vi "Main_agv.vi"() -> ()   [LabVIEW 2019]
doc: "Self driving example made by ybbaek for ERP42."
uses:
  Ctrl/state.ctl
  Ctrl/agv_config.ctl
  Ctrl/gnss_config.ctl
  <vilib>/userDefined/High Color/IMAQdx.ctl
  Ctrl/system_hw.ctl
  C:/Users/WEGO/Documents/GitHub/Ycar/LabVIEW/Gmap/dll/GMap.NET.WindowsForms.dll
  Gmap/dll/GMap.NET.WindowsForms.dll
  Ctrl/joystick cfg.ctl
  Ctrl/joystick_opval.ctl
  Ctrl/error_cluster.ctl
  Ctrl/imu-cfg.ctl
  Ctrl/ledmatrix_data.ctl
  Ctrl/cmd_common.ctl
  Ctrl/log_buffq.ctl
  Ctrl/agv_cmd_v.ctl
  Ctrl/obstacle_info.ctl
  Ctrl/pid-in-params.ctl
  Ctrl/waypoint_buf.ctl
  Ctrl/cmd_imu.ctl
  Ctrl/gps-databuf.ctl
  Gmap/gmap_fgv-cmd.ctl
  Ctrl/sound-data.ctl
  Subvi/log/logfile-name.vi
  Subvi/global_setting.vi
  Ctrl/pid-cfg.ctl
panel:
  out "mode out":enum16{"joystick", "self-driving"}(ring)
  out "joystick":cluster{"X":dbl, "Y":dbl}[](graph)
  out "Mem":dbl(slide) scale=0.0..16000000000.0 scale format="%_1p"
  out "CPU":dbl(slide) scale=0.0..100.0 scale format="%_1f"
  out "Map_Total":T1(graph)=[{"stop pt array out"=[]}, {"stop pt array out"=[]}, {"stop pt array out"=[{"X"=4530998.623923, "Y"=6178450.805513}, {"X"=4530998.538097, "Y"=6178450.804328}, {"X"=4530998.436351, "Y"=6178450.81696}, {"X"=4530998.335494, "Y"=6178450.839631}, {"X"=4530998.287734, "Y"=6178450.881083}, {"X"=4530998.369203, "Y"=6178451.026592}, {"X"=4530998.616099, "Y"=6178451.104199}, {"X"=4530998.899282, "Y"=6178451.204366}, {"X"=4530999.432829, "Y"=6178451.227778}, {"X"=4530999.994657, "Y"=6178451.1834}, {"X"=4531000.491916, "Y"=6178451.184252}, {"X"=4531000.925496, "Y"=6178451.240374}, {"X"=4531001.380332, "Y"=6178451.342912}, {"X"=4531001.869676, "Y"=6178451.447932}, {"X"=4531002.371383, "Y"=6178451.498979}, {"X"=4531002.905819, "Y"=6178451.53243}, {"X"=4531003.356208, "Y"=6178451.584774}, {"X"=4531003.754389, "Y"=6178451.628375}, {"X"=4531004.172048, "Y"=6178451.698315}, {"X"=4531004.577345, "Y"=6178451.822228}, {"X"=4531004.966722, "Y"=6178451.959958}, {"X"=4531005.304781, "Y"=6178452.098985}, {"X"=4531005.558793, "Y"=6178452.256904}, {"X"=4531005.663298, "Y"=6178452.468907}, {"X"=4531005.735073, "Y"=6178452.698506}, {"X"=4531005.808628, "Y"=6178452.948183}, {"X"=4531005.871598, "Y"=6178453.271912}, {"X"=4531005.874357, "Y"=6178453.496547}, {"X"=4531005.809877, "Y"=6178453.736296}, {"X"=4531005.695859, "Y"=6178453.997419}, {"X"=4531005.514602, "Y"=6178454.273656}, {"X"=4531005.263439, "Y"=6178454.53489}, {"X"=4531004.89372, "Y"=6178454.812535}, {"X"=4531004.439065, "Y"=6178455.099032}, {"X"=4531003.810977, "Y"=6178455.363081}, {"X"=4531003.261601, "Y"=6178455.548003}, {"X"=4531002.709556, "Y"=6178455.702809}, {"X"=4531002.017699, "Y"=6178455.827609}, {"X"=4531001.45765, "Y"=6178455.892064}, {"X"=4531000.845393, "Y"=6178455.947777}, {"X"=4531000.166788, "Y"=6178456.028643}, {"X"=4530999.390883, "Y"=6178456.172335}, {"X"=4530998.64593, "Y"=6178456.278353}, {"X"=4530997.881499, "Y"=6178456.358033}, {"X"=4530997.114399, "Y"=6178456.407596}, {"X"=4530996.505611, "Y"=6178456.308947}, {"X"=4530996.309053, "Y"=6178456.025486}, {"X"=4530996.530954, "Y"=6178455.627487}, {"X"=4530996.701536, "Y"=6178455.230783}, {"X"=4530996.904848, "Y"=6178454.816484}, {"X"=4530997.126748, "Y"=6178454.418484}, {"X"=4530997.382268, "Y"=6178454.012928}, {"X"=4530997.604168, "Y"=6178453.614928}, {"X"=4530997.677451, "Y"=6178453.281051}, {"X"=4530997.953338, "Y"=6178452.911871}, {"X"=4530998.350449, "Y"=6178452.556397}, {"X"=4530998.886482, "Y"=6178452.22089}, {"X"=4530999.254422, "Y"=6178451.923168}, {"X"=4530999.465739, "Y"=6178451.599218}, {"X"=4530999.52666, "Y"=6178451.319314}, {"X"=4530999.555832, "Y"=6178451.261562}, {"X"=4530999.57442, "Y"=6178451.277862}, {"X"=4530999.57531, "Y"=6178451.287901}, {"X"=4530999.561169, "Y"=6178451.321796}, {"X"=4530999.562948, "Y"=6178451.341874}, {"X"=4530999.582425, "Y"=6178451.368212}, {"X"=4530999.584204, "Y"=6178451.38829}, {"X"=4530999.552364, "Y"=6178451.415925}, {"X"=4530999.520524, "Y"=6178451.44356}]}]
  out "Error cluster out":T2
  out "State":T3
  out "loop count out":T4
  out "Time info":T5={"Time_total"=2.602255344390869, "Time_run"=0.0, "Time_wait"=2.602255344390869} {"Time_total" format="%.1f"; "Time_run" format="%.1f"; "Time_wait" format="%.1f"}
  in  "ybbaek copyright":string="Made by ybbaek"
  in  "Tab_main":enum32{"Main UI", "Config"}(tab)
  in  "sel driving mode":bool
  out "point all":T6(graph)
  out "Image_color":T7(plugin-control)
  out "LiDAR Display":T8(graph)=[{"Array out"=[{"x"=0.0, "y"=0.0}, {"x"=1.1593565889372284, "y"=0.6693548387096749}, {"x"=0.0, "y"=0.0}, {"x"=-1.0549176217638336, "y"=0.8241919750327333}]}, {"Array out"=[{"x"=0.2522907528348065, "y"=-0.9679098297538085}, {"x"=0.24254936669439534, "y"=-0.9773529581047719}, {"x"=0.2311466414632541, "y"=-0.9780573756893088}, {"x"=0.22013509908304701, "y"=-0.9790570913647973}, {"x"=0.21252085784239536, "y"=-0.9958252595118947}, {"x"=0.20354094471094616, "y"=-1.0117287600074318}, {"x"=0.19216973869870496, "y"=-1.0136956417132665}, {"x"=0.18000768331848416, "y"=-1.0144024331823698}, {"x"=0.16839887138747095, "y"=-1.0130996101644822}, {"x"=0.13425505056226478, "y"=-1.0262556121154827}, {"x"=0.1235875841313941, "y"=-1.0321271041148787}, {"x"=0.11209282841873203, "y"=-1.0392221900619176}, {"x"=0.05343374521033363, "y"=-1.046887241957221}, {"x"=0.04042794561687843, "y"=-1.043467126321284}, {"x"=0.029222649738115388, "y"=-1.0400895570777948}, {"x"=0.017036653056079584, "y"=-1.0411106160983312}, {"x"=0.005134519873165823, "y"=-1.0459873979669507}, {"x"=-0.006314508810403322, "y"=-1.052481057776568}, {"x"=-0.0010110708384152129, "y"=0.0007350073194916896}, {"x"=0.001141793129326704, "y"=-0.000508732198531145}, {"x"=3.2663755682368802, "y"=-0.2409423369298104}, {"x"=3.2682974720954157, "y"=-0.3156008299968731}, {"x"=0.2578445921202276, "y"=-0.9633398822919943}, {"x"=0.24825106355708415, "y"=-0.9697280079706766}, {"x"=0.23807482826060586, "y"=-0.978709833734536}, {"x"=0.2259487186744975, "y"=-0.977475185889316}, {"x"=0.21158377943464465, "y"=-1.0172282459114828}, {"x"=0.19914944525971545, "y"=-1.0156596371091782}, {"x"=0.1865928320916569, "y"=-1.0144828066616085}, {"x"=0.17483503646380183, "y"=-1.0125161529697693}, {"x"=0.16287079283932476, "y"=-1.0140030102716113}, {"x"=0.12952794839316292, "y"=-1.0293827085127565}, {"x"=0.11787284633583305, "y"=-1.0345566947232467}, {"x"=0.10740206219988796, "y"=-1.0409740856693848}, {"x"=0.059584119729109916, "y"=-1.0493096457557736}, {"x"=0.047185684852639714, "y"=-1.0479382191450923}, {"x"=0.034928532242850446, "y"=-1.0409141403763138}, {"x"=0.022959984335812273, "y"=-1.0392464044293341}, {"x"=0.011371685382685006, "y"=-1.0424379764626561}, {"x"=-0.000572277070893853, "y"=-1.0492498439356348}, {"x"=-0.012356443381401225, "y"=-1.0536775506799803}]}, {"Array out"=[]}, {"Array out"=[]}, {"Array out"=[]}]
  out "Pid dt":u32=100
  out "heaading_ui":dbl
  out "Distance_left":dbl format="%.1f"
  out "Dis_gap":dbl format="%.1f"
  out "pro_all":u8(slide) scale=0.0..100.0
  out "pro_curr":dbl(slide)=nan scale=0.0..1.0
  out "stop time":dbl(slide)=2.7272372245788574 scale=0.0..5.0
  in  "gmap zoom":dbl(slide) scale=3.0..20.0
  in  "GMapControl":refnum<k24>(container)
  out "Map_Current":T9(graph)=[{"heading_curr "=[]}, {"heading_curr "=[]}, {"heading_curr "=[{"x"=0.0, "y"=0.0}, {"x"=0.0, "y"=0.0}, {"x"=0.0, "y"=0.0}, {"x"=0.0, "y"=0.0}, {"x"=0.0, "y"=0.0}, {"x"=0.0, "y"=0.0}]}, {"heading_curr "=[]}, {"heading_curr "=[{"x"=0.0, "y"=0.0}, {"x"=0.0, "y"=0.0}]}, {"heading_curr "=[{"x"=0.0, "y"=0.0}, {"x"=0.0, "y"=0.0}]}, {"heading_curr "=[{"x"=0.0, "y"=0.0}, {"x"=3.6739403974420594e-16, "y"=6.0}]}, {"heading_curr "=[{"x"=0.0, "y"=0.0}, {"x"=3.6739403974420594e-16, "y"=6.0}]}]
  in  "imu reset M":bool
  out "latlong_Gmap":cluster{dbl, dbl} {"?" format="%.8f"; "?" format="%.8f"}
  out "latlong_GNSS":cluster{dbl, dbl} {"?" format="%.8f"; "?" format="%.8f"}
  in  "SetMapProvider":u16(ring)=12 items=["None", "OpenStreetMap", "OpenStreet4UMap", "OpenCycleMap", "OpenCycleLandscapeMap", "OpenCycleTransportMap", "OpenStreetMapQuest", "OpenStreetMapQuestSattelite", "OpenStreetMapQuestHybrid", "OpenSeaMapHybrid", "WikiMapiaMap", "BingMap", "BingSatelliteMap", "BingHybridMap", "YahooMap", "YahooSatelliteMap", "YahooHybridMap", "GoogleMap", "GoogleSatelliteMap", "GoogleHybridMap", "GoogleTerrainMap", "GoogleChinaMap", "GoogleChinaSatelliteMap", "GoogleChinaHybridMap", "GoogleChinaTerrainMap", "GoogleKoreaMap", "GoogleKoreaSatelliteMap", "GoogleKoreaHybridMap", "NearMap", "NearSatelliteMap", "NearHybridMap", "OviMap", "OviSatelliteMap", "OviHybridMap", "OviTerrainMap", "YandexMap", "YandexSatelliteMap", "YandexHybridMap", "LithuaniaMap", "Lithuania 2.5d Map", "LithuaniaOrtoFotoMap", "LithuaniaOrtoFotoMapOld", "LithuaniaHybridMap", "LithuaniaHybridMapOld", "LithuaniaTOP50", "LatviaMap", "MapBender, WMS demo", "TurkeyMap", "CloudMade, Demo", "SpainMap", "CzechMap", "CzechSatelliteMap", "CzechHybridMap", "CzechTuristMap", "CzechHistoryMap", "ArcGIS_Imagery_World_2D_Map", "ArcGIS_ShadedRelief_World_2D_Map", "ArcGIS_StreetMap_World_2D_Map", "ArcGIS_Topo_US_2D_Map", "ArcGIS_World_Physical_Map", "ArcGIS_World_Shaded_Relief_Map", "ArcGIS_World_Street_Map", "ArcGIS_World_Terrain_Base_Map", "ArcGIS_World_Topo_Map", "ArcGIS_DarbAE_Q2_2011_NAVTQ_Eng_V5_MapProvider"]
  in  "PinDropMrkr":T10(ring)=enum."red_dot" caption="Pin Drop Marker"
  in  "zoom-center":bool
  in  "Zoom":bool
  in  "Scale_map":dbl(slide)=5.0 min=0.0 scale=5.0..100.0
  in  "ratio":dbl=10.0 format="%#_13g"
  in  "full scale":bool
  out "Steer_PID2":T11(graph)={"output high"=42.0, "output low"=10.0, "output"=0.0}
  in  "Speed":dbl(slide)=33.0 min=0.0 max=255.0 scale=0.0..255.0
  in  "set state value":T3
  in  "state change":bool
  out "network check":bool
  in  "Tap_config":T12(tab)=enum."GNSS Gmap"
  out "Mem usage":dbl(slide) scale=0.0..20000.0 scale format="%_1f"
  out "CPU Usage":dbl(slide) scale=0.0..100.0 scale format="%_1f"
  out "Mem Usage 2":string
  in  "HW info":T13={"AGV"=enum."Ycar", "Lidar 1"=enum."RPLidar A2", "Lidar 2"=enum."none", "GPS"=enum."none", "Camera"=enum."MS LifeCam", "Joystick"=enum."joystick", "sound"=enum."none", "IMU"=enum."none", "Led"=enum."none"}
  out "CPU Chart":dbl(graph)
  out "Mem  Chart":dbl(graph)
  in  "AGV-2":enum32{"Status"}(tab)
  out "batt":dbl(slide) scale=26.0..29.0
  out "AGV velocity Chart":T14(graph)
  out "System Feedback":T15
  in  "AGV cfg":T16={"Port"="COM6", "limits"={"speed limits"={"max"=100.0, "min"=0.0}, "steer limits"={"width"=40.0, "offset"=8.0}}, "dir"=FALSE}
  in  "Lookahead cfg":T17={"lookahead points"=64.0, "lookahead distance"=2.0} {"lookahead distance" format="%.1f"; "lookahead points" format="%#_13g"}
  in  "State machine cfg":T18={" turn steer speed"=0.0, "move speed"=0.0, "slow down factor"=1.0, "adjust angle margin"=0.0} {"slow down factor" min=1.0}
  out "Slide":cluster{dbl, dbl, dbl}(slide) scale=0.0..1.0
  out "Stop point count":u32(slide) scale=-1.0..60.0
  in  "Tab_Lidar-config":enum32{"VLP16", "Tim571", "RPLiar A123"}(tab)=enum."RPLiar A123"
  in  "TIM571 cfg":T19 {"h range" scale=-180.0..180.0}
  in  "RPLidar cfg":T20={"port"="COM3", "dt"=4, "cicle"=28, "speed"=500, "rate"=115200} {"speed" scale=100.0..1000.0}
  out "LiDAR Display for cfg":T8(graph)=[{"Array out"=[{"x"=0.0, "y"=0.0}, {"x"=0.7193398003386512, "y"=0.6946583704589973}, {"x"=0.0, "y"=0.0}, {"x"=-0.9271838545667873, "y"=0.37460659341591224}]}, {"Array out"=[]}, {"Array out"=[]}, {"Array out"=[]}, {"Array out"=[]}]
  in  "lidat setting tab":enum32{"Range", "Limit", "Graph"}(tab)
  in  "VLP16 cfg":T21={"h range"={46, -68}, "v range"={8, -4}} {"v range" scale=-15.0..15.0; "h range" scale=-180.0..180.0}
  in  "Obstacle limit cfg":cluster{"Range":dbl, "Points":u16}={"Range"=1.0, "Points"=110} {"Points" min=10 max=5000 scale=10.0..100.0; "Range" min=0.5 max=200.0 scale=0.5..20.0}
  in  "Lidar graph scale":dbl(slide)=1.0 min=1.0 scale=1.0..10.0
  in  "PID cfg":T22={"PID gains"={"proportional gain (Kc)"=0.01, "integral time (Ti, min)"=0.0, "derivative time (Td, min)"=0.0}, "PID limits"={"output high"=40.0, "output low"=15.0}, "dt_pid"=100} {"PID limits"."output low" format="%.3f"; "PID limits"."output high" format="%.3f"; "PID gains"."derivative time (Td, min)" format="%.4f"; "PID gains"."integral time (Ti, min)" format="%.4f"; "PID gains"."proportional gain (Kc)" format="%.4f"}
  out "Steer_PID1":T11(graph)={"output high"=40.0, "output low"=15.0, "output"=0.0}
  out "Image_binary 2":T7(plugin-control)
  in  "GNSS cfg":T23={"Port"="COM10", "heading select"="", "PwrPak7_mode select"=[], "rate"=115200}
  in  "gmap-dt2":u32=1000
  in  "gmap-dt1":u32=200
  out "Lon_GM":dbl format="%.9f"
  out "Lat_GM":dbl format="%.9f"
  out "Lat_DbClk":dbl format="%.9f"
  out "Lon_DbClk":dbl format="%.9f"
  out "Image_binary":T7(plugin-control)
  out "Image_gray":T7(plugin-control)
  in  "Tab vision-setting":enum32{"Port ", "Config", "camera attrib"}(tab)
  in  "camera cfg":cluster{"Port":T24, "Camera file":path}={"Port"="cam1", "Camera file"=path "C:/AGV/Config/camera/MS_LifeCam_30fps_160x120.icd"}
  in  "Vison cfg":T25 {"Threshold Range"."Upper value" scale=0.0..255.0; "Threshold Range"."Lower value" scale=0.0..255.0}
  in  "camera_attrib":cluster{"brightness":u16, "ExposureTimeAbs":dbl}={"brightness"=0, "ExposureTimeAbs"=15000.0} {"brightness" scale=0.0..10.0; "ExposureTimeAbs" scale=0.0..30000.0}
  in  "IMU cfg":T26={"Port"="COM10", "offset"=0.0, "rate"=115200}
  out "IMU out":T27 {"gyr" format="%.2f"; "mag" format="%.2f"; "acc" format="%.2f"; "angle" format="%.2f"}
  out "dir":picture
  out "heading_cfg":dbl format="%.1f"
  in  "imu reset":bool
  out "ang":dbl[](array[numeric])
  out "Deg-gap_heading-wpt":dbl format="%.1f"
  in  "config save":bool
  in  "config load":bool
  in  "config_file-name":string="user1"
  out "error out":errorcluster
  out "log path":string
  in  "waypoint files cfg":T28={"Waypoint array"=[{"sel"=TRUE, "inv"=FALSE, "path"=path "C:/AGV/Config/waypoint/wpt_shinsung-circle_20201004-1.txt"}]}
  out "Total map cfg":T29(graph)=[{"ref waypt 0703 A \ngoal point start"=[]}, {"ref waypt 0703 A \ngoal point start"=[{"X"=4530998.623923, "Y"=6178450.805513}, {"X"=4530998.538097, "Y"=6178450.804328}, {"X"=4530998.436351, "Y"=6178450.81696}, {"X"=4530998.335494, "Y"=6178450.839631}, {"X"=4530998.287734, "Y"=6178450.881083}, {"X"=4530998.369203, "Y"=6178451.026592}, {"X"=4530998.616099, "Y"=6178451.104199}, {"X"=4530998.899282, "Y"=6178451.204366}, {"X"=4530999.432829, "Y"=6178451.227778}, {"X"=4530999.994657, "Y"=6178451.1834}, {"X"=4531000.491916, "Y"=6178451.184252}, {"X"=4531000.925496, "Y"=6178451.240374}, {"X"=4531001.380332, "Y"=6178451.342912}, {"X"=4531001.869676, "Y"=6178451.447932}, {"X"=4531002.371383, "Y"=6178451.498979}, {"X"=4531002.905819, "Y"=6178451.53243}, {"X"=4531003.356208, "Y"=6178451.584774}, {"X"=4531003.754389, "Y"=6178451.628375}, {"X"=4531004.172048, "Y"=6178451.698315}, {"X"=4531004.577345, "Y"=6178451.822228}, {"X"=4531004.966722, "Y"=6178451.959958}, {"X"=4531005.304781, "Y"=6178452.098985}, {"X"=4531005.558793, "Y"=6178452.256904}, {"X"=4531005.663298, "Y"=6178452.468907}, {"X"=4531005.735073, "Y"=6178452.698506}, {"X"=4531005.808628, "Y"=6178452.948183}, {"X"=4531005.871598, "Y"=6178453.271912}, {"X"=4531005.874357, "Y"=6178453.496547}, {"X"=4531005.809877, "Y"=6178453.736296}, {"X"=4531005.695859, "Y"=6178453.997419}, {"X"=4531005.514602, "Y"=6178454.273656}, {"X"=4531005.263439, "Y"=6178454.53489}, {"X"=4531004.89372, "Y"=6178454.812535}, {"X"=4531004.439065, "Y"=6178455.099032}, {"X"=4531003.810977, "Y"=6178455.363081}, {"X"=4531003.261601, "Y"=6178455.548003}, {"X"=4531002.709556, "Y"=6178455.702809}, {"X"=4531002.017699, "Y"=6178455.827609}, {"X"=4531001.45765, "Y"=6178455.892064}, {"X"=4531000.845393, "Y"=6178455.947777}, {"X"=4531000.166788, "Y"=6178456.028643}, {"X"=4530999.390883, "Y"=6178456.172335}, {"X"=4530998.64593, "Y"=6178456.278353}, {"X"=4530997.881499, "Y"=6178456.358033}, {"X"=4530997.114399, "Y"=6178456.407596}, {"X"=4530996.505611, "Y"=6178456.308947}, {"X"=4530996.309053, "Y"=6178456.025486}, {"X"=4530996.530954, "Y"=6178455.627487}, {"X"=4530996.701536, "Y"=6178455.230783}, {"X"=4530996.904848, "Y"=6178454.816484}, {"X"=4530997.126748, "Y"=6178454.418484}, {"X"=4530997.382268, "Y"=6178454.012928}, {"X"=4530997.604168, "Y"=6178453.614928}, {"X"=4530997.677451, "Y"=6178453.281051}, {"X"=4530997.953338, "Y"=6178452.911871}, {"X"=4530998.350449, "Y"=6178452.556397}, {"X"=4530998.886482, "Y"=6178452.22089}, {"X"=4530999.254422, "Y"=6178451.923168}, {"X"=4530999.465739, "Y"=6178451.599218}, {"X"=4530999.52666, "Y"=6178451.319314}, {"X"=4530999.555832, "Y"=6178451.261562}, {"X"=4530999.57442, "Y"=6178451.277862}, {"X"=4530999.57531, "Y"=6178451.287901}, {"X"=4530999.561169, "Y"=6178451.321796}, {"X"=4530999.562948, "Y"=6178451.341874}, {"X"=4530999.582425, "Y"=6178451.368212}, {"X"=4530999.584204, "Y"=6178451.38829}, {"X"=4530999.552364, "Y"=6178451.415925}, {"X"=4530999.520524, "Y"=6178451.44356}]}]
  in  "test waypoint":bool
  in  "stop points edit":bool
  in  "stop point config":cluster{"distance":dbl, "time":dbl}={"distance"=1.0, "time"=5.0}
  in  "Joystick cfg":T30={"Type"=enum."Logitech F710", "steer limit"={"min"=10.0, "max"=42.0, "scale"=0.0, "offset"=0.0}, "speed limit"={"min"=10.0, "max"=42.0, "pwm max"=0.0}, "ID"=0, "joystick max"=0.0}
  out "opval":T31
  out "pid limit ref":cluster{dbl, dbl}
  out "receive buff out":string
  in  "sound cfg":T32={"id"=0, "music folder"=path "C:/AGV/Config/sound/music", "engine"=path "C:/AGV/Config/sound/lock.wav", "warning"=path "C:/AGV/Config/sound/lock.wav", "msg"=path "C:/AGV/Config/sound/lock.wav", "music"=path "C:/AGV/Config/sound/lock.wav", "unlock"=path "C:/AGV/Config/sound/lock.wav"}
  in  "ledmatrix cfg":T33={"ip"="", "data"="", "Port"="COM6", "time"=""}
  out "LiDAR img":T7(plugin-control)
  in  "pause-resume":bool
  in  "Checking":bool
  in  "start-stop":bool
  in  "close":bool
  in  "Status detail":string="\r\n00:38:31.5 - System start \r\n"
  # "Status main"
  # "64\n  5"
  # "254\n     0"
  # "40\n  8"
  # "4\n44\n444"
  # "X, Y, Z / roll, pitch, yaw"
  # "<Xbox>\njoy max: 32767\nsteer min 10 / scale 16\nsteer max 42 / offset 26\nspeed min 10 / pwm max 255\nspeed max 200"
  # "<F710>\njoy max: 32767\nsteer min 10 / scale 20 (-20)\nsteer max 42 / offset 30\nspeed min 10 / pwm max 255\nspeed max 200              -255"
  # "SRC (Self driving RC Car)"
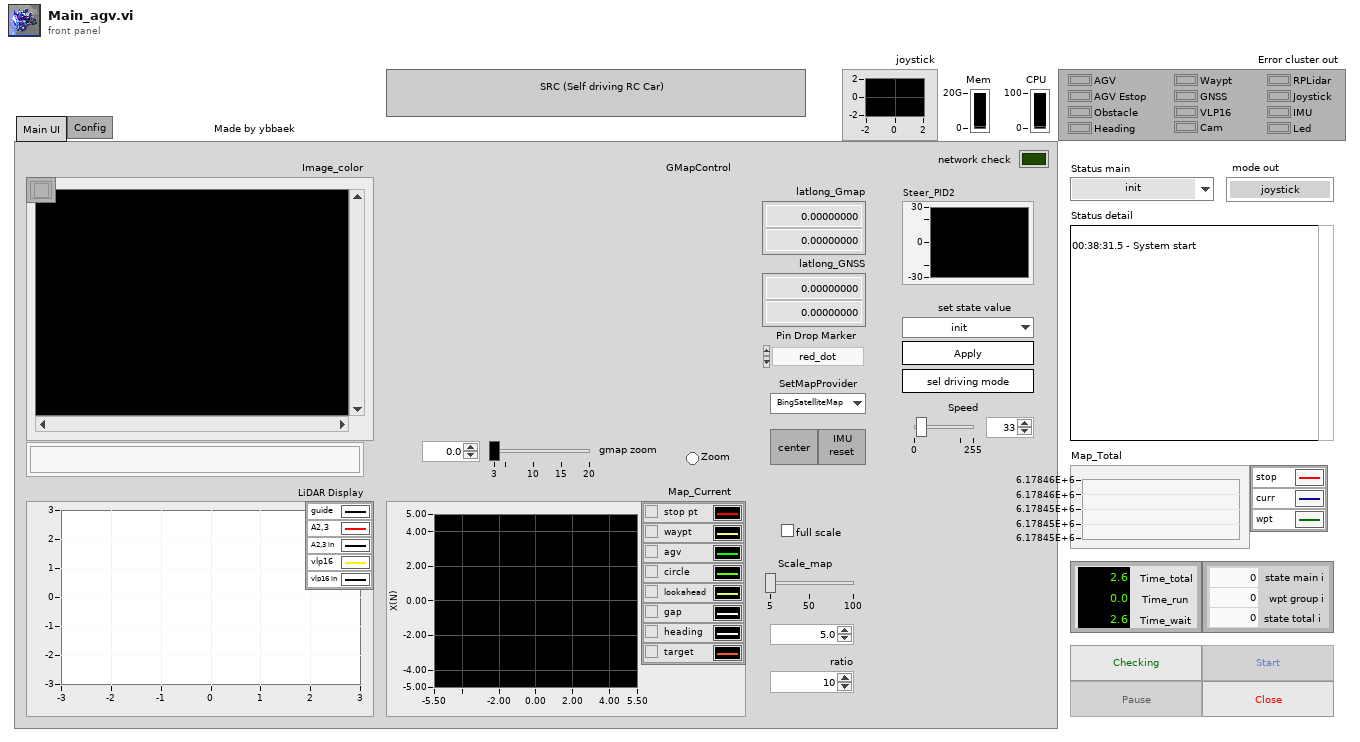
[diagram p1: front panel]
types:
  T1 = cluster{"stop pt array out":cluster{"X":dbl, "Y":dbl}[]}[]
  T2 = typedef "error_cluster.ctl" = cluster{"AGV":u8, "AGV Estop":u8, "Obstacle":u8, "Heading":u8, "Waypt":u8, "GNSS":u8, "VLP16":u8, "Cam":u8, "RPLidar":u8, "Joystick":u8, "IMU":u8, "Led":u8}
  T3 = typedef "state.ctl" = enum16{"init", "Test circular track", "start point", "start heading adjust", "wait before start", "stop point check", "stop point start", "end point", "entering ending point", "move", "move heading adjust"}
  T4 = cluster{"wpt group i":i32, "state total i":i32, "state main i":i32}
  T5 = cluster{"Time_total":dbl, "Time_run":dbl, "Time_wait":dbl}
  T6 = cluster{"Points-2":cluster{"X":sgl, "Y":sgl}[]}[]
  T7 = typedef "IMAQ Image.ctl" = refnum<image>
  T8 = cluster{"Array out":cluster{"x":dbl, "y":dbl}[]}[]
  T9 = cluster{"heading_curr ":cluster{"x":dbl, "y":dbl}[]}[]
  T10 = enum16{"none", "arrow", "blue", "blue_small", "blue_dot", "blue_pushpin", "brown_small", "gray_small", "green", "green_small", "green_dot", "green_pushpin", "green_big_go", "yellow", "yellow_small", "yellow_dot", "yellow_big_pause", "yellow_pushpin", "lightblue", "lightblue_dot", "lightblue_pushpin", "orange", "orange_small", "orange_dot", "pink", "pink_dot", "pink_pushpin", "purple", "purple_small", "purple_dot", "purple_pushpin", "red", "red_small", "red_dot", "red_pushpin", "red_big_stop", "black_small", "white_small"}
  T11 = cluster{"output high":dbl, "output low":dbl, "output":dbl}
  T12 = enum32{"System", "AGV", "LIDAR", "PID", "GNSS Gmap", "Vision", "IMU", "File", "Waypoint", "Joystick", "Network", "Sound", "Led display", "Etc"}
  T13 = typedef "system_hw.ctl" = cluster{"AGV":enum16{"none", "ERP42", "Scout", "Ycar"}, "Lidar 1":enum16{"none", "VLP16", "TIM571", "RPLidar A2", "RPLidar A3"}, "Lidar 2":enum16{"none", "VLP16", "TIM571", "RPLidar A2", "RPLidar A3"}, "GPS":enum16{"none", "F9P", "M8P", "PwrPak7", "19X HVS"}, "Camera":enum16{"none", "C920", "C922", "GT1290C", "MS LifeCam"}, "Joystick":enum16{"none", "joystick"}, "sound":enum16{"none", "speaker"}, "IMU":enum16{"none", "MW-AHRSv1"}, "Led":enum16{"none", "LedMatrix 8x32"}}
  T14 = cluster{"Linear Velocity (m/s)":dbl, "Angular Velocity (rad/s)":dbl, "Battery Voltage":dbl}
  T15 = cluster{"state":string, "Mode":u8, "Battery V":dbl, "error High":u8, "error Low":u8}
  T16 = typedef "agv_config.ctl" = cluster{"Port":refnum<visa-resource-name>, "limits":cluster{"speed limits":cluster{"max":dbl, "min":dbl}, "steer limits":cluster{"width":dbl, "offset":dbl}}, "dir":bool}
  T17 = cluster{"lookahead points":dbl, "lookahead distance":dbl}
  T18 = cluster{" turn steer speed":dbl, "move speed":dbl, "slow down factor":dbl, "adjust angle margin":dbl}
  T19 = cluster{"TIM571 IP":string, "h range":cluster{i16, i16}}
  T20 = cluster{"port":refnum<visa-resource-name>, "dt":u32, "cicle":u8, "speed":u16, "rate":u32}
  T21 = cluster{"h range":cluster{i16, i16}, "v range":cluster{i8, i8}}
  T22 = cluster{"PID gains":cluster{"proportional gain (Kc)":dbl, "integral time (Ti, min)":dbl, "derivative time (Td, min)":dbl}, "PID limits":cluster{"output high":dbl, "output low":dbl}, "dt_pid":u32}
  T23 = typedef "gnss_config.ctl" = cluster{"Port":refnum<visa-resource-name>, "heading select":string, "PwrPak7_mode select":string[], "rate":u32}
  T24 = typedef "IMAQdx.ctl" = refnum<k21>
  T25 = cluster{"Clamp Settings":cluster{"Contrast":i32, "Filter width":i32, "Steepness":i32, "Subsampling Ratio":u32, "Show Search Area":bool, "Show Search Lines":bool, "Show Edges Found":bool, "Show Result":bool}, "Threshold Range":cluster{"Lower value":sgl, "Upper value":sgl}, "N of Erosion 1":i32, "N of Erosion 2":i32}
  T26 = typedef "imu-cfg.ctl" = cluster{"Port":refnum<visa-resource-name>, "offset":dbl, "rate":u32}
  T27 = cluster{"angle":dbl[], "acc":dbl[], "mag":dbl[], "gyr":dbl[]}
  T28 = cluster{"Waypoint array":cluster{"sel":bool, "inv":bool, "path":path}[]}
  T29 = cluster{"ref waypt 0703 A \ngoal point start":cluster{"X":dbl, "Y":dbl}[]}[]
  T30 = typedef "joystick cfg.ctl" = cluster{"Type":enum16{"Logitech F710", "Xbox"}, "steer limit":cluster{"min":dbl, "max":dbl, "scale":dbl, "offset":dbl}, "speed limit":cluster{"min":dbl, "max":dbl, "pwm max":dbl}, "ID":i32, "joystick max":dbl}
  T31 = typedef "joystick_opval.ctl" = cluster{"curr":u32, "last":u32}
  T32 = cluster{"id":u32, "music folder":path, "engine":path, "warning":path, "msg":path, "music":path, "unlock":path}
  T33 = typedef "ledmatrix_data.ctl" = cluster{"ip":string, "data":string, "Port":refnum<visa-resource-name>, "time":string}
  T34 = cluster{"VLP16 cfg":refnum<vi>, "TIM571 cfg":refnum<vi>, "PID cfg":refnum<vi>, "AGV cfg":refnum<vi>, "GNSS cfg":refnum<vi>, "camera cfg":refnum<vi>, "ybbaek copyright":refnum<vi>, "Obstacle limit cfg":refnum<vi>, "State machine cfg":refnum<vi>, "Lookahead cfg":refnum<vi>, "waypoint files cfg":refnum<vi>, "Vison cfg":refnum<vi>, "RPLidar cfg":refnum<vi>, "point all":refnum<vi>, "HW info":refnum<vi>, "Joystick cfg":refnum<vi>, "GMapControl":refnum<vi>, "IMU cfg":refnum<vi>, "ledmatrix cfg":refnum<vi>}
  T35 = enum16{"Config Save", "Config Load", "LastRUN Save", "LastRUN Load"}
  T36 = typedef "cmd_common.ctl" = enum16{"read", "write"}
  T37 = cluster{"Name":string, "Color":u32, "Style":u8, "Point Style":u8, "Name Visible":bool, "Allow Drag":bool, "Annotation Mode":u32, "Plot":i32, "Index":i32, "Position":cluster{"X":dbl, "Y":dbl}, "X Scale":u32, "Y Scale":u32, "Show Arrow":bool, "Lock Name":bool, "Plot Area":i32, "Label Offset":cluster{"X":dbl, "Y":dbl}}
  T38 = enum8{"Enabled", "Disabled", "Disabled and Grayed Out"}
  T39 = typedef "log_buffq.ctl" = enum16{"create", "write", "read", "close"}
  T40 = typedef "agv_cmd_v.ctl" = enum16{"write limit", "init stop", "write", "read"}
  T41 = cluster{"zoom":dbl, "dt clear":u32, "dt add ":u32, "PinDropMrkr":enum16{"none", "arrow", "blue", "blue_small", "blue_dot", "blue_pushpin", "brown_small", "gray_small", "green", "green_small", "green_dot", "green_pushpin", "green_big_go", "yellow", "yellow_small", "yellow_dot", "yellow_big_pause", "yellow_pushpin", "lightblue", "lightblue_dot", "lightblue_pushpin", "orange", "orange_small", "orange_dot", "pink", "pink_dot", "pink_pushpin", "purple", "purple_small", "purple_dot", "purple_pushpin", "red", "red_small", "red_dot", "red_pushpin", "red_big_stop", "black_small", "white_small"}, "zoom n center":bool}
  T42 = cluster{"VLP16 cfg":cluster{"h range":cluster{i16, i16}, "v range":cluster{i8, i8}}, "TIM571 cfg":cluster{"IP":string, "h range":cluster{i16, i16}}, "AGV cfg":T16, "GPS cfg":cluster{"Port":refnum<visa-resource-name>, "heading select":string, "PwrPak7_mode select":string[], "rate":u32}, "PID cfg":cluster{"PID gains":cluster{"proportional gain (Kc)":dbl, "integral time (Ti, min)":dbl, "derivative time (Td, min)":dbl}, "PID limits":cluster{"output high":dbl, "output low":dbl}, "dt pid":u32}, "Lookahead cfg":cluster{"lookahead pts n":dbl, "lookahead distance":dbl}, "Obstacle limit range":cluster{"RL range":dbl, "Point limit":u16}, "State machine parameter":cluster{"angle adjust limit":dbl}, "waypoint group":cluster{"Waypoint array":cluster{"sel":bool, "inv":bool, "path":path}[]}, "State machine cfg":cluster{" turn angular speed":dbl, "move linear speed":dbl, "decrease factor linear speed":dbl, "adjust angle margin":dbl}, "camera cfg":cluster{"Port":T24, "Camera file":path}, "ROI-clamp":cluster{"Global Rectangle":i32[], "Contours":cluster{"Contour Type":u32, "ROI Type":u32, "Points":i32[]}[]}, "x-center":dbl, "Image Size":cluster{"x":i32, "y":i32}, "Angle deg":sgl, "Vison cfg":cluster{"Clamp Settings":cluster{"Contrast":i32, "Filter width":i32, "Steepness":i32, "Subsampling Ratio":u32, "Show Search Area":bool, "Show Search Lines":bool, "Show Edges Found":bool, "Show Result":bool}, "Range":cluster{"Lower value":sgl, "Upper value":sgl}, "N of Erosion 1":i32, "N of Erosion 2":i32}, "RPLidar cfg":cluster{"port":refnum<visa-resource-name>, "dt":u32, "update":u8, "speed":u16, "rate ":u32}, "HW info":T13, "Joystick cfg":T30, "IMU cfg":T26, "ledmatrix cfg":T33}
  T43 = cluster{"Name":string, "Color":u32, "Style":u8, "Point Style":u8, "Name Visible":bool, "Allow Drag":bool, "Annotation Mode":u32, "Plot":i32, "Index":i32, "Position":cluster{"X":dbl, "Y":dbl}, "X Scale":u32, "Y Scale":u32, "Show Arrow":bool, "Lock Name":bool, "Plot Area":i32, "Label Offset":cluster{"X":dbl, "Y":dbl}}[]
  T44 = cluster{"Global Rectangle":i32[], "Contours":cluster{"Contour Type":u32, "ROI Type":u32, "Points":i32[]}[]}
  T45 = cluster{"Lat_GM":refnum<vi>, "Lon_GM":refnum<vi>, "Lat_DbClk":refnum<vi>, "Lon_DbClk":refnum<vi>, "gmap zoom":refnum<vi>, "PinDropMrkr":refnum<vi>}
  T46 = typedef "obstacle_info.ctl" = enum16{"init", "read", "obstacle status in", "write limit", "inrange pt-n"}
  T47 = typedef "pid-in-params.ctl" = enum16{"read", "write"}
  T48 = typedef "waypoint_buf.ctl" = enum16{"clear", "write", "read"}
  T49 = typedef "pid-cfg.ctl" = enum16{"read", "write pid gain", "write pid limit", "pid dt"}
  T50 = typedef "gps-databuf.ctl" = enum16{"read", "write"}
  T51 = typedef "cmd_imu.ctl" = enum16{"ini", "write", "read"}
  T52 = typedef "gmap_fgv-cmd.ctl" = enum16{"marker type change", "save_image", "coll of points", "zoom n center markers", "add overlay reference", "read", "zoom", "set position by keyword", "set map provider", "map provider update", "create", "add marker", "clear marker", "close"}
  T53 = enum16{"check", "unlock", "engine", "warning", "msg", "music"}
  T54 = typedef "sound-data.ctl" = cluster{"FN":enum16{"check", "unlock", "engine", "warning", "msg", "music"}, "Data":variant}
  T55 = cluster{"total time":dbl, "run time":dbl, "wait time":dbl}
  T56 = cluster{"deg_agv-lookahead":dbl, "deg_waypoint":dbl, "deg_gap":dbl, "deg_target":dbl, "pid output":dbl, "dis-gap":dbl, "deg_agv-center":dbl}
  T57 = cluster{"lookahead pt n":dbl, "lookahead distance":dbl}
  T58 = cluster{"System Feedback":cluster{"system state":string, "Control Mode":u8, "Battery Voltage":dbl, "error code High":u8, "error code Low":u8}, "Motion Feedback":cluster{"Linear Velocity (m/s)":dbl, "Angular Velocity (rad/s)":dbl}}
  T59 = cluster{"system state":string, "Control Mode":u8, "Battery Voltage":dbl, "error code High":u8, "error code Low":u8}
  T60 = cluster{"Linear Velocity (m/s)":dbl, "Angular Velocity (rad/s)":dbl}
  T61 = cluster{"start point":cluster{"x":dbl, "y":dbl}, "stop point":cluster{"x":dbl, "y":dbl}}
  T62 = cluster{"progress_curr":dbl, "progress_all":dbl, "distance_left":dbl, "distance_all":dbl}
  T63 = cluster{"output high":dbl, "output low":dbl, "pid output":dbl}
  T64 = cluster{"total time":dbl, "run time":dbl, "pause time":dbl}
  T65 = cluster{"rawdata":string, "GPS Data":cluster{"Latitude":cluster{"Valid?":bool, "Latitude (Deg)":dbl}, "Longitude":cluster{"Valid?":bool, "Longitude (Deg)":dbl}, "Height":cluster{"Valid?":bool, "Height (m)":dbl}, "Undulation":cluster{"Valid?":bool, "Undulation(m)":dbl}, "North Vel":cluster{"Valid?":bool, "North Vel (m/s)":dbl}, "East Vel":cluster{"Valid?":bool, "East Vel (m/s)":dbl}, "Up Vel":cluster{"Valid?":bool, "Up Vel (m/s)":dbl}, "Roll":cluster{"Valid?":bool, "Roll (degrees)":dbl}, "Pitch":cluster{"Valid?":bool, "Pitch (degrees)":dbl}, "Azimuth":cluster{"Valid?":bool, "Azimuth (degrees)":dbl}, "Lat deviation":cluster{"Valid?":bool, "Lat deviation (m)":dbl}, "Long deviation":cluster{"Valid?":bool, "Long deviation (m)":dbl}, "Height deviation":cluster{"Valid?":bool, "Height deviation (m)":dbl}, "North vel deviation":cluster{"Valid?":bool, "North vel deviation (m/s)":dbl}, "East vel deviation":cluster{"Valid?":bool, "East vel deviation (m/s)":dbl}, "Up vel deviation":cluster{"Valid?":bool, "Up vel deviation (m/s)":dbl}, "Roll deviation":cluster{"Valid?":bool, "Roll deviation (degrees)":dbl}, "Pitch deviation":cluster{"Valid?":bool, "Pitch deviation (degrees)":dbl}, "Azimuth deviation":cluster{"Valid?":bool, "Azimuth deviation (degrees)":dbl}, "Ext sol status":cluster{"Valid?":bool, "Ext sol status":dbl}}, "Heading":dbl, "utm-1":cluster{"XN":dbl, "YE":dbl}}
  T66 = typedef "mapinfo.ctl" = cluster{"GmapDotNet":refnum<k24>, "mapprovider_info":cluster{"index":i32, "dotnetrefs":refnum<k24>, "Name":string}[]}
  T67 = cluster{"index":i32, "dotnetrefs":refnum<k24>, "Name":string}[]
  T68 = cluster{"index":i32, "dotnetrefs":refnum<k24>, "Name":string}
  T69 = cluster{"gmap zoom":dbl, "gmap-dt1":u32, "gmap-dt2":u32, "PinDropMrkr":enum16{"none", "arrow", "blue", "blue_small", "blue_dot", "blue_pushpin", "brown_small", "gray_small", "green", "green_small", "green_dot", "green_pushpin", "green_big_go", "yellow", "yellow_small", "yellow_dot", "yellow_big_pause", "yellow_pushpin", "lightblue", "lightblue_dot", "lightblue_pushpin", "orange", "orange_small", "orange_dot", "pink", "pink_dot", "pink_pushpin", "purple", "purple_small", "purple_dot", "purple_pushpin", "red", "red_small", "red_dot", "red_pushpin", "red_big_stop", "black_small", "white_small"}, "Zoom":bool}
  T70 = enum16{"none", "VLP16", "TIM571", "RPLidar A2", "RPLidar A3"}
  T71 = enum16{"none", "F9P", "M8P", "PwrPak7", "19X HVS"}
  T72 = enum16{"none", "C920", "C922", "GT1290C", "MS LifeCam"}
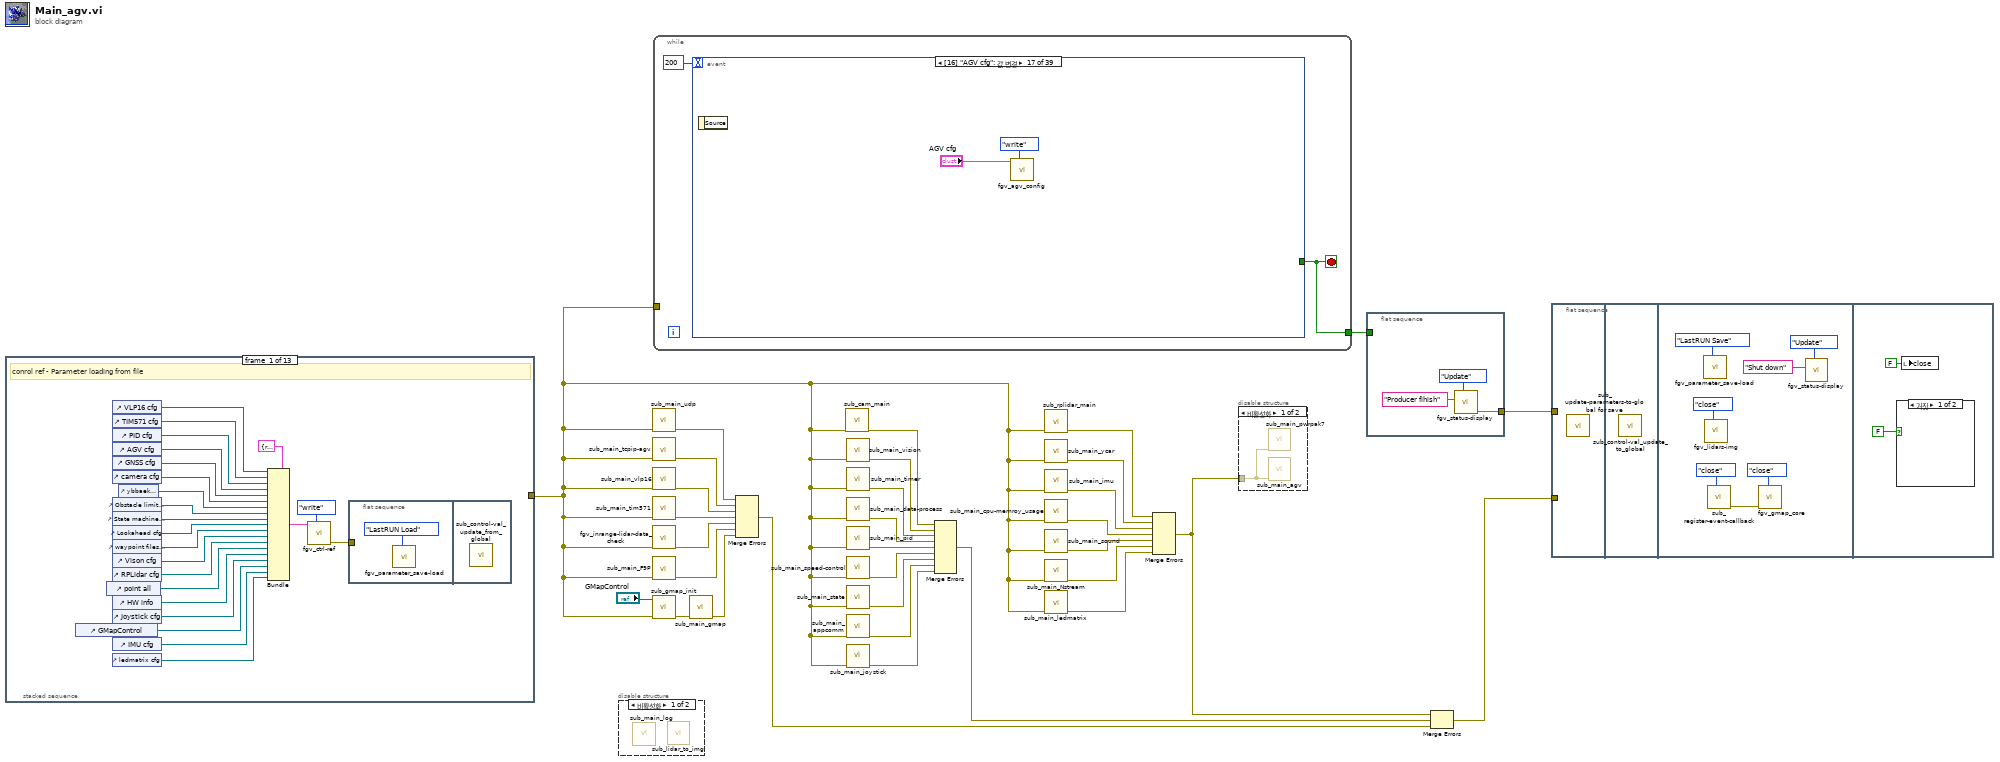
[diagram p0: block diagram]
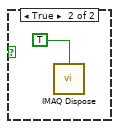
[diagram p4: hidden frame]
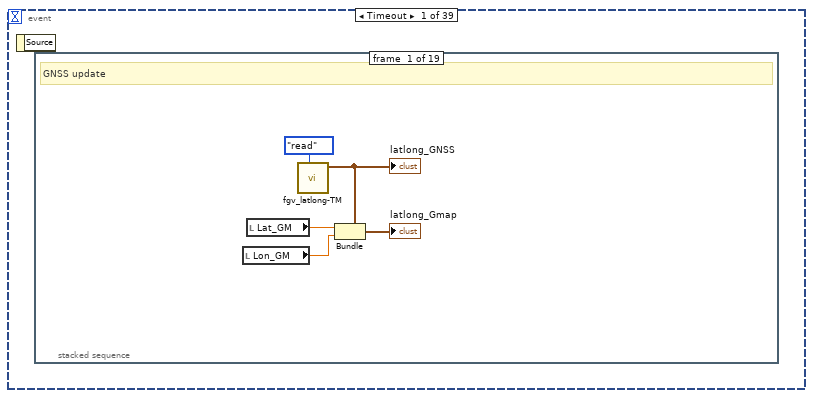
[diagram p5: hidden frame]
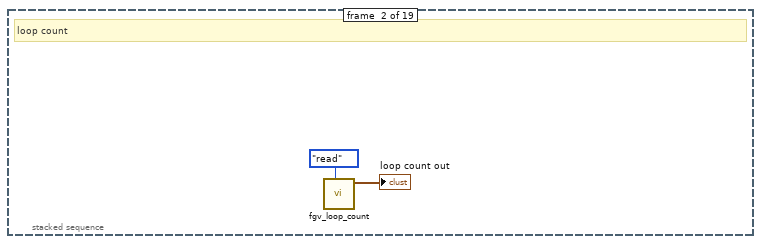
[diagram p6: hidden frame]
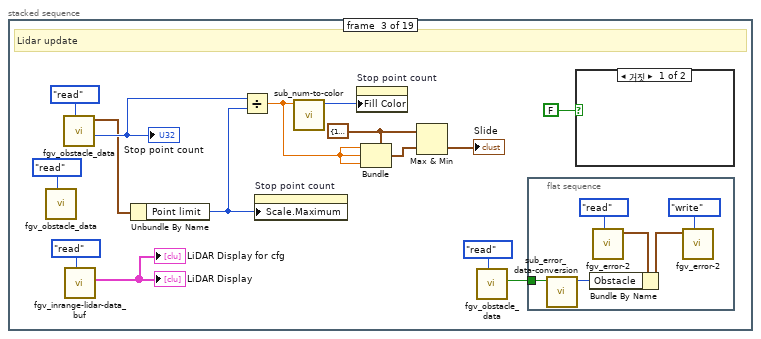
[diagram p7: hidden frame]
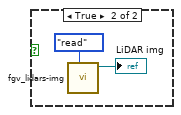
[diagram p8: hidden frame]
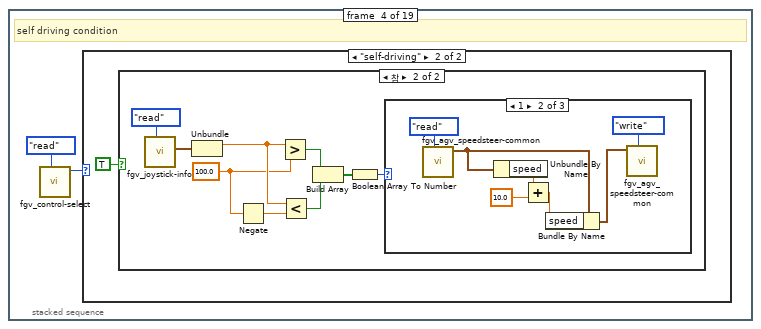
[diagram p9: hidden frame]
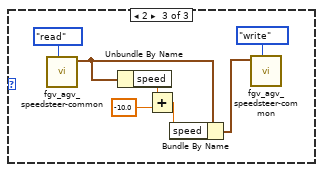
[diagram p13: hidden frame]
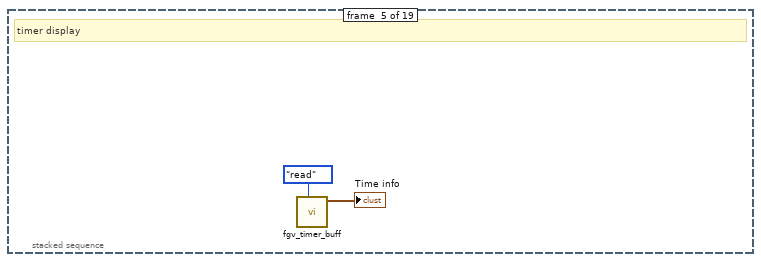
[diagram p14: hidden frame]
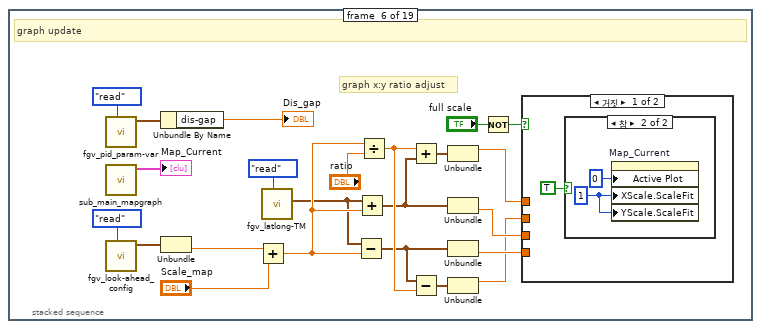
[diagram p15: hidden frame]
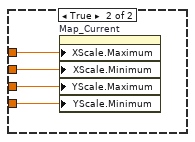
[diagram p17: hidden frame]
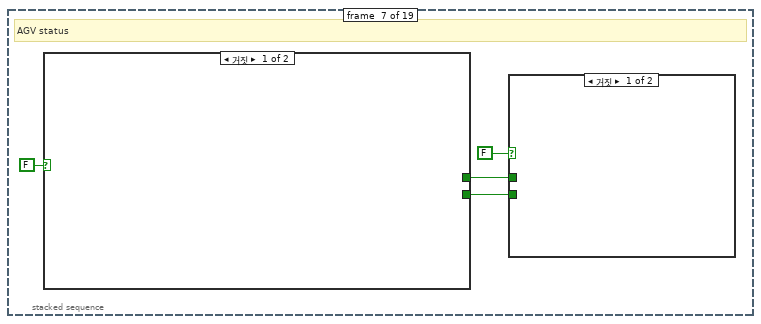
[diagram p18: hidden frame]
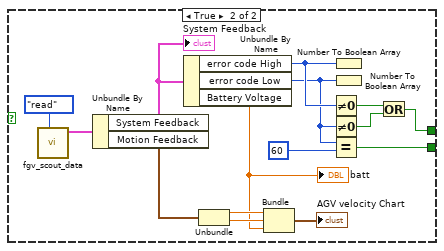
[diagram p19: hidden frame]
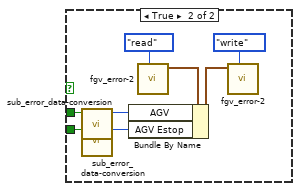
[diagram p20: hidden frame]
diagram:
  n1 = stacked-sequence {
    tunnel: [_ _ _ _ w92 _ _ _ _ _ _ _ _] -> w2
    frame #0 {
      # "conrol ref - Parameter loading from file"
      n2 = control-ref of="GMapControl"() -> (w37:refnum<vi>)
      n3 = control-ref of="point all"() -> (w42:refnum<vi>)
      n4 = control-ref of="VLP16 cfg"() -> (w47:refnum<vi>)
      n5 = control-ref of="TIM571 cfg"() -> (w55:refnum<vi>)
      n6 = control-ref of="PID cfg"() -> (w54:refnum<vi>)
      n7 = control-ref of="AGV cfg"() -> (w53:refnum<vi>)
      n8 = control-ref of="GNSS cfg"() -> (w52:refnum<vi>)
      n9 = control-ref of="camera cfg"() -> (w46:refnum<vi>)
      n10 = control-ref of="Obstacle limit cfg"() -> (w51:refnum<vi>)
      n11 = control-ref of="State machine cfg"() -> (w50:refnum<vi>)
      n12 = control-ref of="Lookahead cfg"() -> (w48:refnum<vi>)
      n13 = control-ref of="waypoint files cfg"() -> (w49:refnum<vi>)
      n14 = control-ref of="Vison cfg"() -> (w45:refnum<vi>)
      n15 = control-ref of="RPLidar cfg"() -> (w43:refnum<vi>)
      n16 = control-ref of="HW info"() -> (w41:refnum<vi>)
      n17 = control-ref of="Joystick cfg"() -> (w39:refnum<vi>)
      n18 = control-ref of="IMU cfg"() -> (w36:refnum<vi>)
      n19 = control-ref of="ledmatrix cfg"() -> (w35:refnum<vi>)
      n20 = control-ref of="ybbaek copyright"() -> (w44:refnum<vi>)
      n21 = Bundle(cluster=T34 {"VLP16 cfg"=refnum, "TIM571 cfg"=refnum, "PID cfg"=refnum, "AGV cfg"=refnum, "GNSS cfg"=refnum, "camera cfg"=refnum, "ybbaek copyright"=refnum, "Obstacle limit cfg"=refnum, "State machine cfg"=refnum, "Lookahead cfg"=refnum, "waypoint files cfg"=refnum, "Vison cfg"=refnum, "RPLidar cfg"=refnum, "point all"=refnum, "HW info"=refnum, "Joystick cfg"=refnum, "GMapControl"=refnum, "IMU cfg"=refnum, "ledmatrix cfg"=refnum} ("클러스터"), "VLP16 cfg"=w47, "TIM571 cfg"=w55, "PID cfg"=w54, "AGV cfg"=w53, "GNSS cfg"=w52, "camera cfg"=w46, "ybbaek copyright"=w44, "Obstacle limit cfg"=w51, "State machine cfg"=w50, "Lookahead cfg"=w48, "waypoint files cfg"=w49, "Vison cfg"=w45, "RPLidar cfg"=w43, "point all"=w42, "HW info"=w41, "Joystick cfg"=w39, "GMapControl"=w37, "IMU cfg"=w36, "ledmatrix cfg"=w35) -> (w34:T34)
      n22 = call "fgv_ctrl-ref.vi"("cmd"=enum16{"write", "read"}."write", "ref"=w34) -> ("error out"=w38:errorcluster)  [unwired: 8 in, 1 out]
      n23 = flat-sequence {
        tunnel: w38 -> [_]
        frame #0 {
          n24 = call "fgv_parameter_save-load.vi"("ctl"=T35."LastRUN Load") -> ()  [unwired: 9 in, 2 out]
        }
        frame #1 {
          n25 = call "sub_control-val_update_from_global.vi"() -> ()  [unwired: 12 in]
        }
      }
    }
    frame #1 {
      # "log init"
      n26 = flat-sequence {
        frame #0 {
          n27 = call "sub_log_fine-name.vi"() -> ("log path"=→"log path":string)  [unwired: 11 in]
        }
        frame #1 {
          n28 = disable-structure shown="비활성화" {
            frame Disabled {
              n29 = global read "global_setting.vi" "Settings"() -> (w62:T42)
              n30 = Flatten To XML(anything=w62) -> (xml string=w61:string)
              n31 = call "sub_log_basic.vi"("desc"=w61, "Title"="log_settings") -> ()  [unwired: 9 in, 1 out]
            }
            frame Enabled {
            }
          }
          n32 = global read "logfile-name.vi" "logfile_name"() -> (w59:string)
          n33 = call "sub_log_basic.vi"("desc"=w59, "Title"="Log path") -> ("error out"=→"error out":errorcluster)  [unwired: 9 in]
        }
        frame #2 {
          n34 = call "sub_check-ip.vi"() -> ("ip output"=w64:string, "standard output"=w69:string)  [unwired: 10 in]
          n35 = call "sub_log_basic.vi"("desc"=w69, "Title"="ip addr") -> ()  [unwired: 9 in, 1 out]
          n36 = disable-structure shown="비활성화" {
            disable-tunnel: w64 -> [w71 _]
            frame Disabled {
              n37 = call "fgv_ledmatrix_config.vi"("cmd"=cmd_common."read") -> ("data out"=w73:T33)  [unwired: 10 in]
              n38 = Bundle By Name(cluster=w73, "ip"=w71) -> (w72:T33)
              n39 = call "fgv_ledmatrix_config.vi"("cmd"=cmd_common."write", "data"=w72) -> ()  [unwired: 9 in, 1 out]
            }
            frame Enabled {
            }
          }
          n40 = call "fgv_system_info.vi"("cmd"=enum16{"read", "write"}."read") -> ("info_out"=w66:cluster{"ip":string})  [unwired: 10 in]
          n41 = Bundle By Name(cluster=w66, "ip"=w64) -> (w65:cluster{"ip":string})
          n42 = call "fgv_system_info.vi"("cmd"=enum16{"read", "write"}."write", "info"=w65) -> ()  [unwired: 9 in, 1 out]
        }
      }
    }
    frame #2 {
      w76 = FALSE ("close")
      w78 = T38."Disabled and Grayed Out" ("비활성화")
      # "etc"
      n43 = case shown="참" FALSE {
        frame False {
        }
        frame True {
          w79 = TRUE ("Name Visible")
          n44 = Bundle By Name(cluster=T37 {"Name"="", "Color"=0, "Style"=0, "Point Style"=0, "Name Visible"=FALSE, "Allow Drag"=FALSE, "Annotation Mode"=0, "Plot"=0, "Index"=0, "Position"={"X"=0.0, "Y"=0.0}, "X Scale"=0, "Y Scale"=0, "Show Arrow"=TRUE, "Lock Name"=FALSE, "Plot Area"=0, "Label Offset"={"X"=0.0, "Y"=0.0}} ("원소"), "Color"=u32 0, "Name Visible"=w79, "Lock Name"=w79) -> (w82:T37)
          n45 = Build Array(w82) -> (w83:T43)
          n46 = property on="Map_Total" class="XYGraph (엄격한)"("AnntList"=w83) -> ()  [unwired: 2 in, 2 out]
        }
      }
      n47 = local write "close"(w76) -> ()
      n48 = local write "start-stop"(w76) -> ()
      n49 = property on="start-stop" class="Bool (엄격한)"("DisabledEnum"=w78) -> ()  [unwired: 2 in, 2 out]
      n50 = property on="pause-resume" class="Bool (엄격한)"("DisabledEnum"=w78) -> ()  [unwired: 2 in, 2 out]
    }
    frame #3 {
      # "display monitor"
      n51 = flat-sequence {
        frame #0 {
          n52 = control-ref of="Status detail"() -> (w88:refnum<vi>)
          n53 = call "fgv_status-display.vi"("Mode"=enum16{"Initial", "Update", "Clear"}."Initial", "System Log"=w88) -> ("error out"=w87:errorcluster)  [unwired: 9 in]
          n54 = call "fgv_status-display.vi"("Mode"=enum16{"Initial", "Update", "Clear"}."Update", "error in"=w87, "title"="System start" ("String in 1")) -> ()  [unwired: 8 in, 1 out]
        }
        frame #1 {
          n55 = global read "logfile-name.vi" "logfile_name"() -> (w89:string)
          n56 = call "fgv_status-display.vi"("Mode"=enum16{"Initial", "Update", "Clear"}."Update", "title"=w89) -> ()  [unwired: 9 in, 1 out]
        }
      }
    }
    frame #4 {
      # "Log in account"
      n57 = case shown="거짓" FALSE {
        tunnel: [T38."Enabled" ("비활성화") w95] -> w91
        frame False {
        }
        frame True {
          n58 = call "login simple.vi"() -> ("pass - fail"=w96:bool)  [unwired: 11 in]
          n59 = case shown="거짓" w96 {
            tunnel: [T38."Disabled and Grayed Out" ("비활성화") T38."Enabled" ("비활성화")] -> w95
            frame False {
            }
            frame True {
            }
          }
        }
      }
      n60 = property on="Checking" class="Bool"("DisabledEnum"=w91) -> (error out=w92:errorcluster)  [unwired: 2 in, 1 out]
    }
    frame #5 {
      # "total map update"
      n61 = call "fgv_waypoint_total.vi"("cmd"=enum16{"write", "read"}."read") -> ("waypoint total out"=w101:cluster{"waypt":cluster{"X":dbl, "Y":dbl}[]}[])  [unwired: 10 in]
      n62 = for {
        shift-right: [w103] -> w102
        shift-left: T29 [] -> [w104]
        tunnel: w101 -> [w105] mode=indexing
        n63 = Build Array (concatenate)(w104, w105) -> (w103:cluster{"waypt":cluster{"X":dbl, "Y":dbl}[]}[])
      }
      n64 = local write "Map_Total"(w102) -> ()
    }
    frame #6 {
      # "hw prod cons q creation"
      n65 = disable-structure shown="비활성화" {
        frame Disabled {
          n66 = call "fgv_q_tim571.vi"("cmd"=enum16{"create", "write", "read", "close"}."create") -> ()  [unwired: 9 in, 2 out]
          n67 = call "fgv_q_vlp16.vi"("cmd"=enum16{"create", "write", "read", "close"}."create") -> ()  [unwired: 9 in, 2 out]
          n68 = call "fgv_q_agv.vi"("cmd"=enum16{"create", "write", "read", "close"}."create") -> ()  [unwired: 9 in, 2 out]
          n69 = call "fgv_erp42_q.vi"("cmd"=enum16{"create", "write", "read", "close"}."create") -> ()  [unwired: 9 in, 2 out]
          n70 = call "fgv_erp42mini-232_q.vi"("cmd"=enum16{"create", "write", "read", "close"}."create") -> ()  [unwired: 9 in, 2 out]
          n71 = call "fgv_q_PwrPak7.vi"("cmd"=enum16{"create", "write", "read", "close"}."create") -> ()  [unwired: 9 in, 2 out]
        }
        frame Enabled {
        }
      }
      n72 = call "fgv_control-select.vi"("cmd"=cmd_common."write", "mode"=enum16{"joystick", "self-driving"}."joystick") -> ()  [unwired: 9 in, 1 out]
      n73 = call "fgv_rplidar_232_q.vi"("cmd"=enum16{"create", "write", "read", "close"}."create") -> ()  [unwired: 9 in, 2 out]
      n74 = call "fgv_sound_q.vi"("cmd"=enum16{"create", "write", "read", "close"}."create") -> ()  [unwired: 9 in, 2 out]
      n75 = call "fgv_ledmatrix_q.vi"("cmd"=enum16{"create", "write", "read", "close"}."create") -> ()  [unwired: 9 in, 2 out]
      n76 = call "fgv_pc_cam_q.vi"("cmd"=enum16{"create", "write", "read", "close"}."create") -> ()  [unwired: 9 in, 2 out]
      n77 = call "fgv_F9P_q.vi"("cmd"=enum16{"create", "write", "read", "close"}."create") -> ()  [unwired: 9 in, 2 out]
      n78 = call "fgv_ycar_q.vi"("cmd"=enum16{"create", "write", "read", "close"}."create") -> ()  [unwired: 9 in, 2 out]
      n79 = call "fgv_q_joystick.vi"("cmd"=enum16{"create", "write", "read", "close"}."create") -> ()  [unwired: 9 in, 2 out]
      n80 = call "fgv_imu_q_pro-con.vi"("cmd"=enum16{"create", "write", "read", "close"}."create") -> ()  [unwired: 9 in, 2 out]
    }
    frame #7 {
      # "not using"
      # "fgv q"
      n81 = disable-structure shown="활성화" {
        frame Disabled {
          n82 = call "fgv_erp42_data.vi"("cmd"=enum16{"init", "read", "write"}."init") -> ()  [unwired: 8 in, 3 out]
        }
        frame Enabled {
        }
      }
      n83 = call "fgv_remote_conn-check.vi"("cmd"=enum16{"write", "read"}."write", "conn"=FALSE) -> ()  [unwired: 9 in, 1 out]
      n84 = call "fgv_stop-point_databuf.vi"("cmd"=enum16{"clear", "write", "read"}."clear") -> ()  [unwired: 9 in, 2 out]
      n85 = call "fgv_local-stop_agv.vi"("cmd"=enum16{"ini", "read", "stop"}."ini") -> ()  [unwired: 10 in, 1 out]
      n86 = call "fgv_global-stop.vi"("cmd"=enum16{"init", "stop", "read"}."init") -> ()  [unwired: 10 in, 1 out]
      n87 = call "fgv_joystick-info.vi"("init"=enum16{"enable", "init", "read", "write"}."init") -> ()  [unwired: 7 in, 4 out]
      n88 = call "fgv_lane_slope-info.vi"("cmd"=enum16{"ini", "read", "write"}."ini") -> ()  [unwired: 8 in, 3 out]
      n89 = call "fgv_error-2.vi"("cmd"=enum16{"init", "read", "write"}."init") -> ()  [unwired: 9 in, 2 out]
      n90 = call "fgv_logbuff_q.vi"("cmd"=log_buffq."create") -> ()  [unwired: 9 in, 2 out]
      n91 = call "fgv_loop_count.vi"("cmd"=enum16{"init", "read", "write"}."init") -> ()  [unwired: 9 in, 2 out]
      n92 = call "fgv_system_state.vi"("cmd"=enum16{"init", "read", "write"}."init") -> ()  [unwired: 9 in, 2 out]
      n93 = call "fgv_lidars-img.vi"("cmd"=enum16{"create", "read", "close"}."create") -> ()  [unwired: 10 in, 1 out]
      n94 = call "sub_system_pause-condition.vi"("cmd"=enum16{"pause", "go", "read"}."pause") -> ()  [unwired: 10 in, 1 out]
      n95 = call "sub_hw-err-checking.vi"("cmd"=enum16{"write", "read", "init"}."init") -> ()  [unwired: 10 in, 1 out]
      n96 = call "fgv_lidars-databuf.vi"("cmd"=enum16{"ini img arr", "write", "read"}."ini img arr") -> ()  [unwired: 9 in, 2 out]
      n97 = call "fgv_hw-err.vi"("cmd"=enum16{"ini", "read", "write"}."ini") -> ()  [unwired: 10 in, 1 out]
    }
    frame #8 {
      # "agv"
      n98 = call "fgv_agv_cmd-val.vi"("cmd"=agv_cmd_v."init stop") -> ()  [unwired: 9 in, 2 out]
      n99 = call "fgv_agv_speedsteer-common.vi"("cmd"=enum16{"init", "read", "write"}."init") -> ()  [unwired: 10 in, 1 out]
      n100 = disable-structure shown="비활성화" {
        frame Disabled {
          n101 = call "fgv_erp42_opval.vi"("cmd"=enum16{"read", "write", "ini"}."ini") -> ()  [unwired: 10 in, 1 out]
          n102 = call "fgv_erp42mini-opval.vi"("cmd"=enum16{"ini", "read", "wirte"}."ini") -> ()  [unwired: 10 in, 1 out]
          n103 = call "fgv_hw-info.vi"("cmd"=enum16{"write", "read"}."write") -> ()  [unwired: 10 in, 1 out]
        }
        frame Enabled {
        }
      }
      n104 = case shown="참" FALSE {
        frame False {
        }
        frame True {
        }
      }
    }
    frame #9 {
      # "way point"
      n105 = call "fgv_waypoint_config.vi"("cmd"=enum16{"read", "write"}."read") -> ("waypoint files cfg out"=w156:T28)  [unwired: 10 in]
      n106 = call "sub_waypoints_upload.vi"("waypoint group"=w156) -> ("waypt error"=w145:bool, "waypoint all"=w157:cluster{"XY 그래프":cluster{"X":dbl, "Y":dbl}[]}[])  [unwired: 9 in]
      n107 = call "fgv_waypoint_total.vi"("cmd"=enum16{"write", "read"}."write", "waypoint total in"=w157) -> ("waypoint total out"=w152:cluster{"waypt":cluster{"X":dbl, "Y":dbl}[]}[])  [unwired: 9 in]
      n108 = call "sub_error_data-conversion.vi"("error status"=w145) -> ("error conversion out"=w146:u8)  [unwired: 9 in, 1 out]
      n109 = Build Array (concatenate)(cluster{"stop pt array out":cluster{dbl, dbl}[]} {"stop pt array out"=[]} ("출력 클러스터"), w152) -> (w151:cluster{"waypt":cluster{"X":dbl, "Y":dbl}[]}[])
      n110 = call "fgv_error-2.vi"("cmd"=enum16{"init", "read", "write"}."read") -> ("Error cluster out"=w149:T2)  [unwired: 9 in, 1 out]
      n111 = Bundle By Name(cluster=w149, "Waypt"=w146) -> (w150:T2)
      n112 = local write "Total map cfg"(w151) -> ()
      n113 = call "fgv_error-2.vi"("cmd"=enum16{"init", "read", "write"}."write", "Error cluster"=w150) -> ()  [unwired: 8 in, 2 out]
    }
    frame #10 {
      # "stop point"
      n114 = call "fgv_stop-point_config.vi"("cmd"=enum16{"read", "write"}."write", "config value"="stop point config") -> ()  [unwired: 9 in, 1 out]
      n115 = call "fgv_timer_stop-point.vi"("cmd"=enum16{"check", "start", "pause"}."start") -> ()  [unwired: 8 in, 3 out]
      n116 = call "fgv_stop-point_databuf.vi"("cmd"=enum16{"clear", "write", "read"}."clear") -> ()  [unwired: 9 in, 2 out]
    }
    frame #11 {
      # "vision"
      n117 = call "fgv_imgbuf_raw.vi"("cmd"=enum16{"create", "close", "write", "read"}."create") -> ()  [unwired: 9 in, 2 out]
      n118 = call "fgv_imgbuf_processing.vi"("cmd"=enum16{"create", "close", "write", "read"}."create") -> ()  [unwired: 9 in, 2 out]
      n119 = call "fgv_imgbuf_binary.vi"("cmd"=enum16{"create", "close", "write", "read"}."create") -> ()  [unwired: 9 in, 2 out]
      n120 = call "fgv_clamp_roi.vi"("cmd"=enum16{"init", "read", "write"}."read") -> ("ROI-clamp out"=w162:T44)  [unwired: 10 in]
      n121 = property on="Image_gray" class="ImageControl"("ROI"=w162) -> ()  [unwired: 2 in, 2 out]
    }
    frame #12 {
      n122 = control-ref of="gmap zoom"() -> (w177:refnum<vi>)
      n123 = control-ref of="PinDropMrkr"() -> (w176:refnum<vi>)
      n124 = control-ref of="Lat_GM"() -> (w174:refnum<vi>)
      n125 = control-ref of="Lon_GM"() -> (w173:refnum<vi>)
      n126 = control-ref of="Lat_DbClk"() -> (w172:refnum<vi>)
      n127 = control-ref of="Lon_DbClk"() -> (w171:refnum<vi>)
      n128 = Bundle("Lat_GM"=w174, "Lon_GM"=w173, "Lat_DbClk"=w172, "Lon_DbClk"=w171, "gmap zoom"=w177, "PinDropMrkr"=w176) -> (w170:T45)  [unwired: 1 in]
      n129 = call "fgv_gmap_config.vi"("cmd"=enum16{"read", "write"}."write", "gmap cfg"=T41 {"zoom"=16.0, "dt clear"=40, "dt add "=1000, "PinDropMrkr"=enum."red_big_stop", "zoom n center"=FALSE}) -> ()  [unwired: 8 in, 2 out]
      n130 = call "fgv_ctr-ref_gmap.vi"("cmd"=cmd_common."write", "ref in"=w170) -> ()  [unwired: 9 in, 1 out]
      n131 = call "fgv_ctrl-ref_cluster.vi"("cmd"=enum16{"read", "write"}."write", "ref"=w170) -> ()  [unwired: 9 in, 1 out]
    }
  }
  n132 = disable-structure shown="비활성화" {
    frame Disabled {
      n133 = call "sub_main_log.vi"() -> ()  [unwired: 11 in, 1 out]
      n134 = call "sub_lidar_to_img.vi"() -> ()  [unwired: 11 in, 1 out]
    }
    frame Enabled {
    }
  }
  n135 = call "sub_main_udp.vi"("error in"=w2) -> ("error out"=w30:errorcluster)  [unwired: 10 in]
  n136 = call "sub_main_tcpip-agv.vi"("error in"=w2) -> ("error out"=w29:errorcluster)  [unwired: 10 in]
  n137 = call "sub_main_vlp16.vi"("error in"=w2) -> ("error out"=w28:errorcluster)  [unwired: 10 in]
  n138 = call "sub_main_tim571.vi"("error in"=w2) -> ("error out"=w27:errorcluster)  [unwired: 10 in]
  n139 = call "fgv_inrange-lidar-data_check.vi"("error in"=w2) -> ("error out"=w21:errorcluster)  [unwired: 10 in]
  n140 = call "sub_main_F9P.vi"("error in"=w2) -> ("error out"=w20:errorcluster)  [unwired: 10 in]
  n141 = call "sub_gmap_init.vi"("error in"=w2, "GMapControl"="GMapControl") -> ("error out"=w6:errorcluster)  [unwired: 9 in]
  n142 = while {
    tunnel: w2 -> [_]
    tunnel: [w179] -> w32
    stop <- w179 stop-if-true
    n143 = event shown="[16] \"AGV cfg\": 값 변경" {
      selector: _ -> [_ _ _ _ _ _ _ _ _ _ _ _ _ _ _ _ _ _ _ _ _ _ _ _ _ _ _ _ _ _ _ _ _ _ _ _ _ _ _]
      dyn-events: _ -> [_ _ _ _ _ _ _ _ _ _ _ _ _ _ _ _ _ _ _ _ _ _ _ _ _ _ _ _ _ _ _ _ _ _ _ _ _ _ _]
      timeout: 200 -> [_ _ _ _ _ _ _ _ _ _ _ _ _ _ _ _ _ _ _ _ _ _ _ _ _ _ _ _ _ _ _ _ _ _ _ _ _ _ _]
      tunnel: [_ _ _ _ _ _ _ _ _ _ _ _ _ _ _ _ _ _ _ _ _ _ _ _ _ _ _ _ _ _ _ _ _ _ _ w657 _ _ _] -> w179
      event Timeout {
        n144 = event-data() -> ()  [unwired: 1 in, 1 out]
        n145 = stacked-sequence {
          frame #0 {
            # "GNSS update"
            n146 = local read "Lon_GM"() -> (w183:dbl)
            n147 = local read "Lat_GM"() -> (w182:dbl)
            n148 = call "fgv_latlong-TM.vi"("cmd"=enum16{"write", "read"}."read") -> ("latlong out"=w180:cluster{"lat":dbl, "long":dbl})  [unwired: 9 in, 1 out]
            "latlong_GNSS" <- w180
            n149 = Bundle(cluster=w180, "lat"=w182, "long"=w183) -> (→"latlong_Gmap":cluster{"lat":dbl, "long":dbl})
          }
          frame #1 {
            # "loop count"
            n150 = call "fgv_loop_count.vi"("cmd"=enum16{"init", "read", "write"}."read") -> ("loop count out"=→"loop count out":T4)  [unwired: 9 in, 1 out]
          }
          frame #2 {
            w192 = cluster{dbl, dbl, dbl} {1.0, 0.8, 0.5} ("Slide 2")
            # "Lidar update"
            n151 = call "fgv_obstacle_data.vi"("cmd"=obstacle_info."read") -> ()  [unwired: 7 in, 4 out]
            n152 = call "fgv_obstacle_data.vi"("cmd"=obstacle_info."read") -> ("inrange pt-n out"=w196:u32, "limit out"=w187:cluster{"RL range":dbl, "Point limit":u16})  [unwired: 7 in, 2 out]
            "Stop point count" <- w196
            n153 = call "fgv_inrange-lidar-data_buf.vi"("cmd"=enum16{"read", "write"}."read") -> ("in range data new out"=→"LiDAR Display" →"LiDAR Display for cfg":T8)  [unwired: 9 in, 1 out]
            n154 = Unbundle By Name(w187) -> ("Point limit"=w195:u16)
            n155 = Divide(x=w196, y=w195) -> (x/y=w190:dbl)
            n156 = property on="Stop point count" class="Slide (엄격한)"("Scale.Maximum"=w195) -> ()  [unwired: 2 in, 2 out]
            n157 = call "sub_num-to-color.vi"("ratio"=w190) -> ("color num"=w194:u32)  [unwired: 10 in]
            n158 = property on="Stop point count" class="Slide (엄격한)"("Fill Color"=w194) -> ()  [unwired: 2 in, 2 out]
            n159 = Bundle(cluster=w192, w190, w190, w190) -> (w193:cluster{dbl, dbl, dbl})
            n160 = Max & Min(x=w192, y=w193) -> (min(x,y)=→"Slide":cluster{dbl, dbl, dbl})  [unwired: 1 out]
            n161 = call "fgv_obstacle_data.vi"("cmd"=obstacle_info."read") -> ("obstacle out"=w200:bool)  [unwired: 7 in, 3 out]
            n162 = flat-sequence {
              tunnel: w200 -> [w204]
              frame #0 {
                n163 = call "sub_error_data-conversion.vi"("error status"=w204) -> ("error conversion out"=w205:u8)  [unwired: 9 in, 1 out]
                n164 = call "fgv_error-2.vi"("cmd"=enum16{"init", "read", "write"}."read") -> ("Error cluster out"=w208:T2)  [unwired: 9 in, 1 out]
                n165 = Bundle By Name(cluster=w208, "Obstacle"=w205) -> (w209:T2)
                n166 = call "fgv_error-2.vi"("cmd"=enum16{"init", "read", "write"}."write", "Error cluster"=w209) -> ()  [unwired: 8 in, 2 out]
              }
            }
            n167 = case shown="거짓" FALSE {
              frame False {
              }
              frame True {
                n168 = call "fgv_lidars-img.vi"("cmd"=enum16{"create", "read", "close"}."read") -> ("New Image"=→"LiDAR img":T7)  [unwired: 10 in]
              }
            }
          }
          frame #3 {
            # "self driving condition"
            n169 = call "fgv_control-select.vi"("cmd"=cmd_common."read") -> ("mode out"=w210:enum16{"joystick", "self-driving"})  [unwired: 10 in]
            n170 = case shown="\"self-driving\"" w210 {
              frame "joystick", Default {
              }
              frame "self-driving" {
                n171 = case shown="참" TRUE {
                  frame False {
                  }
                  frame True {
                    w218 = 100.0 ("y")
                    n172 = call "fgv_joystick-info.vi"("init"=enum16{"enable", "init", "read", "write"}."read") -> ("v_val"=w220:cluster{dbl, dbl})  [unwired: 7 in, 3 out]
                    n173 = Unbundle(w220) -> (w219:dbl)  [unwired: 1 out]
                    n174 = Negate(x=w218) -> (-x=w217:dbl)
                    n175 = Greater?(x=w219, y=w218) -> (0:w215:bool)
                    n176 = Less?(x=w219, y=w217) -> (x < y?=w216:bool)
                    n177 = Build Array(w215, w216) -> (w214:bool[])
                    n178 = Boolean Array To Number(Boolean array=w214) -> (number=w213:u32)
                    n179 = case shown="1" w213 {
                      frame 0, Default {
                      }
                      frame 1 {
                        n180 = call "fgv_agv_speedsteer-common.vi"("cmd"=enum16{"init", "read", "write"}."read") -> ("speed-steer out"=w225:cluster{"speed":dbl, "steer":dbl})  [unwired: 10 in]
                        n181 = Unbundle By Name(w225) -> ("speed"=w224:dbl)
                        n182 = Add(x=w224, y=10.0) -> (x+y=w223:dbl)
                        n183 = Bundle By Name(cluster=w225, "speed"=w223) -> (w226:cluster{"speed":dbl, "steer":dbl})
                        n184 = call "fgv_agv_speedsteer-common.vi"("cmd"=enum16{"init", "read", "write"}."write", "speed-steer"=w226) -> ()  [unwired: 9 in, 1 out]
                      }
                      frame 2 {
                        n185 = call "fgv_agv_speedsteer-common.vi"("cmd"=enum16{"init", "read", "write"}."read") -> ("speed-steer out"=w232:cluster{"speed":dbl, "steer":dbl})  [unwired: 10 in]
                        n186 = Unbundle By Name(w232) -> ("speed"=w231:dbl)
                        n187 = Add(x=w231, y=-10.0) -> (x+y=w230:dbl)
                        n188 = Bundle By Name(cluster=w232, "speed"=w230) -> (w233:cluster{"speed":dbl, "steer":dbl})
                        n189 = call "fgv_agv_speedsteer-common.vi"("cmd"=enum16{"init", "read", "write"}."write", "speed-steer"=w233) -> ()  [unwired: 9 in, 1 out]
                      }
                    }
                  }
                }
              }
            }
          }
          frame #4 {
            # "timer display"
            n190 = call "fgv_timer_buff.vi"("cmd"=enum16{"write", "read"}."read") -> ("time_status out"=→"Time info":T55)  [unwired: 10 in]
          }
          frame #5 {
            # "graph x:y ratio adjust"
            # "graph update"
            n191 = call "fgv_pid_param-var.vi"("cmd"=pid-in-params."read") -> ("pid-var_output"=w241:T56)  [unwired: 10 in]
            n192 = call "sub_main_mapgraph.vi"() -> ("graph ui array"=→"Map_Current":T9)  [unwired: 11 in]
            n193 = call "fgv_look-ahead_config.vi"("cmd"=enum16{"read", "write"}."read") -> ("lookahed cfg out"=w256:T57)  [unwired: 10 in]
            n194 = Unbundle By Name(w241) -> ("dis-gap"=→"Dis_gap":dbl)
            n195 = Unbundle(w256) -> ("lookahead distance"=w255:dbl)  [unwired: 1 out]
            n196 = Add(x=w255, y="Scale_map") -> (x+y=w253:dbl)
            n197 = call "fgv_latlong-TM.vi"("cmd"=enum16{"write", "read"}."read") -> ("tm out"=w239:cluster{"YE":dbl, "XN":dbl})  [unwired: 9 in, 1 out]
            n198 = Subtract(x=w239, y=w253) -> (x-y=w249:cluster{"YE":dbl, "XN":dbl})
            n199 = Add(x=w239, y=w253) -> (x+y=w250:cluster{"YE":dbl, "XN":dbl})
            n200 = Divide(x=w253, y="ratio") -> (x/y=w251:dbl)
            n201 = Add(x=w251, y=w250) -> (x+y=w247:cluster{"YE":dbl, "XN":dbl})
            n202 = Subtract(x=w249, y=w251) -> (x-y=w248:cluster{"YE":dbl, "XN":dbl})
            n203 = Unbundle(w247) -> ("YE"=w244:dbl)  [unwired: 1 out]
            n204 = Unbundle(w250) -> ("XN"=w260:dbl)  [unwired: 1 out]
            n205 = Unbundle(w249) -> ("XN"=w259:dbl)  [unwired: 1 out]
            n206 = Unbundle(w248) -> ("YE"=w243:dbl)  [unwired: 1 out]
            n207 = Not(x="full scale") -> (.not. x?=w242:bool)
            n208 = case shown="거짓" w242 {
              tunnel: w260 -> [_ w267]
              tunnel: w259 -> [_ w266]
              tunnel: w244 -> [_ w265]
              tunnel: w243 -> [_ w264]
              frame False {
                n209 = case shown="참" TRUE {
                  frame False {
                  }
                  frame True {
                    w263 = u8 1 ("X Scale.Scale Fit")
                    n210 = property on="Map_Current" class="XYGraph (엄격한)"("Active Plot"=u32 0 ("활성 플롯"), "XScale.ScaleFit"=w263, "YScale.ScaleFit"=w263) -> ()  [unwired: 2 in, 2 out]
                  }
                }
              }
              frame True {
                n211 = property on="Map_Current" class="XYGraph (엄격한)"("XScale.Maximum"=w265, "XScale.Minimum"=w264, "YScale.Maximum"=w267, "YScale.Minimum"=w266) -> ()  [unwired: 2 in, 2 out]
              }
            }
          }
          frame #6 {
            # "AGV status"
            n212 = case shown="거짓" FALSE {
              tunnel: [_ w273] -> w271
              tunnel: [_ w272] -> w270
              frame False {
              }
              frame True {
                n213 = call "fgv_scout_data.vi"("cmd"=enum16{"write", "read"}."read") -> ("agv data out"=w283:T58)  [unwired: 10 in]
                n214 = Unbundle By Name(w283) -> ("System Feedback"=w279:T59, "Motion Feedback"=w278:T60)
                "System Feedback" <- w279
                n215 = Unbundle By Name(w279) -> ("error code High"=w281:u8, "error code Low"=w280:u8, "Battery Voltage"=w274:dbl)
                "batt" <- w274
                n216 = Unbundle(w278) -> ("Linear Velocity (m/s)"=w277:dbl, "Angular Velocity (rad/s)"=w276:dbl)
                n217 = Bundle("Linear Velocity (m/s)"=w277, "Angular Velocity (rad/s)"=w276, "Battery Voltage"=w274) -> (→"AGV velocity Chart":T14)  [unwired: 1 in]
                n218 = Not Equal To 0?(x=w281) -> (x != 0?=w284:bool)
                n219 = Not Equal To 0?(x=w280) -> (x != 0?=w285:bool)
                n220 = Equal?(x=w280, y=u8 60) -> (x = y?=w272:bool)
                n221 = Number To Boolean Array(number=w281) -> ()  [unwired: 1 out]
                n222 = Number To Boolean Array(number=w280) -> ()  [unwired: 1 out]
                n223 = Or(x=w284, y=w285) -> (x .or. y?=w273:bool)
              }
            }
            n224 = case shown="거짓" FALSE {
              tunnel: w271 -> [_ w288]
              tunnel: w270 -> [_ w287]
              frame False {
              }
              frame True {
                n225 = call "sub_error_data-conversion.vi"("error status"=w288) -> ("error conversion out"=w290:u8)  [unwired: 9 in, 1 out]
                n226 = call "sub_error_data-conversion.vi"("error status"=w287) -> ("error conversion out"=w289:u8)  [unwired: 9 in, 1 out]
                n227 = call "fgv_error-2.vi"("cmd"=enum16{"init", "read", "write"}."read") -> ("Error cluster out"=w293:T2)  [unwired: 9 in, 1 out]
                n228 = Bundle By Name(cluster=w293, "AGV"=w290, "AGV Estop"=w289) -> (w294:T2)
                n229 = call "fgv_error-2.vi"("cmd"=enum16{"init", "read", "write"}."write", "Error cluster"=w294) -> ()  [unwired: 8 in, 2 out]
              }
            }
          }
          frame #7 {
            # "distance"
            n230 = call "fgv_waypoint_data.vi"("cmd"=waypoint_buf."read") -> ("start-stop point"=w298:T61)  [unwired: 8 in, 2 out]
            n231 = call "fgv_latlong-TM.vi"("cmd"=enum16{"write", "read"}."read") -> ("tm out"=w295:cluster{"YE":dbl, "XN":dbl})  [unwired: 9 in, 1 out]
            n232 = Unbundle By Name(w298) -> ("stop point"=w297:cluster{"x":dbl, "y":dbl})
            n233 = call "sub_measure_distance.vi"("pt 2"=w295, "pt 1"=w297) -> ("distance"=w296:dbl)  [unwired: 9 in]
            "Distance_left" <- w296
            n234 = flat-sequence {
              tunnel: w296 -> [w302]
              frame #0 {
                n235 = call "fgv_system_progress.vi"("cmd"=enum16{"read", "write"}."read") -> ("progress status out"=w303:T62)  [unwired: 10 in]
                n236 = Bundle By Name(cluster=w303, "distance_left"=w302) -> (w301:T62)
                n237 = call "fgv_system_progress.vi"("cmd"=enum16{"read", "write"}."write", "progress status"=w301) -> ()  [unwired: 9 in, 1 out]
              }
            }
          }
          frame #8 {
            # "system progress"
            n238 = call "fgv_waypoint_curr_index.vi"("cmd"=enum16{"write", "read"}."read") -> ("index out"=w306:i32)  [unwired: 10 in]
            n239 = call "fgv_waypoint_data.vi"("cmd"=waypoint_buf."read") -> ("waypoint out"=w310:cluster{"x":dbl, "y":dbl}[])  [unwired: 8 in, 2 out]
            n240 = Array Size(array=w310) -> (size(s)=w307:i32)
            n241 = Divide(x=w306, y=w307) -> (x/y=w308:dbl)
            "pro_curr" <- w308
            n242 = flat-sequence {
              tunnel: w308 -> [w312]
              frame #0 {
                n243 = call "fgv_system_progress.vi"("cmd"=enum16{"read", "write"}."read") -> ("progress status out"=w316:T62)  [unwired: 10 in]
                n244 = Bundle By Name(cluster=w316, "progress_curr"=w312) -> (w315:T62)
                n245 = call "fgv_system_progress.vi"("cmd"=enum16{"read", "write"}."write", "progress status"=w315) -> ()  [unwired: 9 in, 1 out]
              }
            }
          }
          frame #9 {
            # "PID status"
            n246 = disable-structure shown="비활성화" {
              frame Disabled {
                n247 = call "fgv_pid_cfg-var.vi"("cmd"=pid-cfg."read") -> ()  [unwired: 7 in, 4 out]
              }
              frame Enabled {
              }
            }
            n248 = call "fgv_pid-config.vi"("cmd"=enum16{"read", "write"}."read") -> ("PID cfg out"=w320:T22)  [unwired: 9 in, 1 out]
            n249 = Unbundle By Name(w320) -> ("PID limits"=w319:cluster{"output high":dbl, "output low":dbl})
            n250 = call "fgv_pid_status.vi"("cmd"=cmd_common."read") -> ("dt out"=→"Pid dt":u32, "pid output"=w322:dbl)  [unwired: 8 in, 1 out]
            n251 = Unbundle(w319) -> ("output high"=w324:dbl, "output low"=w323:dbl)
            n252 = Bundle("output high"=w324, "output low"=w323, "pid output"=w322) -> (→"Steer_PID2" →"Steer_PID1":T63)  [unwired: 1 in]
          }
          frame #10 {
            # "state display"
            n253 = call "fgv_control-select.vi"("cmd"=cmd_common."read") -> ("mode out"=→"mode out":enum16{"joystick", "self-driving"})  [unwired: 10 in]
            n254 = call "fgv_system_state.vi"("cmd"=enum16{"init", "read", "write"}."read") -> ("State out"=→"State":T3)  [unwired: 9 in, 1 out]
          }
          frame #11 {
            # "Total map update"
            n255 = call "sub_map-data_all.vi"() -> ("map-data_all"=→"Map_Total":T29)  [unwired: 11 in]
          }
          frame #12 {
            # "Error / network"
            n256 = call "fgv_error-2.vi"("cmd"=enum16{"init", "read", "write"}."read") -> ("Error cluster out"=→"Error cluster out":T2)  [unwired: 9 in, 1 out]
            n257 = call "fgv_remote_conn-check.vi"("cmd"=enum16{"write", "read"}."read") -> ("conn_result"=→"network check":bool)  [unwired: 10 in]
          }
          frame #13 {
            # "stop point display"
            n258 = call "fgv_stop-point_config.vi"("cmd"=enum16{"read", "write"}."read") -> ("config value out"=w336:cluster{"stop distance":dbl, "Stop delay":dbl})  [unwired: 10 in]
            n259 = Unbundle By Name(w336) -> ("Stop delay"=w338:dbl)
            n260 = call "fgv_timer_stop-point.vi"("cmd"=enum16{"check", "start", "pause"}."check", "target time"=w338) -> ("time_status_out"=w340:T64)  [unwired: 7 in, 2 out]
            n261 = property on="stop time" class="Slide (엄격한)"("Scale.Maximum"=w338) -> ()  [unwired: 2 in, 2 out]
            n262 = Unbundle By Name(w340) -> ("total time"=→"stop time":dbl)
          }
          frame #14 {
            # "vision display"
            n263 = call "fgv_imgbuf_raw.vi"("cmd"=enum16{"create", "close", "write", "read"}."read") -> ("Image"=→"Image_color":T7)  [unwired: 9 in, 1 out]
            n264 = call "sub_lane-point_interpolation.vi"("cmd"=enum16{"init", "read", "write"}."read") -> ("graph data"=→"point all":T6)  [unwired: 7 in, 3 out]
            n265 = local read "Tap_config"() -> (w342:T12)
            n266 = case shown="\"Vision\"" w342 {
              frame "System", Default {
              }
              frame "AGV" {
              }
              frame "LIDAR" {
              }
              frame "PID" {
              }
              frame "GNSS Gmap" {
              }
              frame "Vision" {
                n267 = call "fgv_imgbuf_binary.vi"("cmd"=enum16{"create", "close", "write", "read"}."read") -> ("raw image out"=→"Image_binary" →"Image_binary 2":T7)  [unwired: 9 in, 1 out]
                n268 = call "fgv_imgbuf_processing.vi"("cmd"=enum16{"create", "close", "write", "read"}."read") -> ("Image"=→"Image_gray":T7)  [unwired: 9 in, 1 out]
              }
              frame "IMU" {
              }
              frame "File" {
              }
              frame "Waypoint" {
              }
              frame "Joystick" {
              }
              frame "Network" {
              }
              frame "Sound" {
              }
              frame "Etc" {
              }
            }
          }
          frame #15 {
            # "Nsteam joystick"
            n269 = call "fgv_joystick-info.vi"("init"=enum16{"enable", "init", "read", "write"}."read") -> ("opval"=→"opval":T31, "v_val"=w356:cluster{dbl, dbl})  [unwired: 7 in, 2 out]
            n270 = call "fgv_udp_receive-data.vi"("cmd"=enum16{"read", "write"}."read") -> ("receive buff out"=w361:string)  [unwired: 10 in]
            "receive buff out" <- w361
            n271 = Unbundle(w356) -> (w354:dbl, w355:dbl)
            n272 = Match Pattern(string=w361, regular expression="VA=" ("정규식")) -> (after substring=w366:string)  [unwired: 1 in, 3 out]
            n273 = Match Pattern(string=w361, regular expression="VL=" ("정규식")) -> (after substring=w370:string)  [unwired: 1 in, 3 out]
            n274 = Bundle(w355, w354) -> (w353:cluster{dbl, dbl})  [unwired: 1 in]
            n275 = Match Pattern(string=w366, regular expression="," ("정규식")) -> (before substring=w367:string)  [unwired: 1 in, 3 out]
            n276 = Match Pattern(string=w370, regular expression="," ("정규식")) -> (before substring=w369:string)  [unwired: 1 in, 3 out]
            n277 = Fract/Exp String To Number(string=w367) -> (number=w363:dbl)  [unwired: 3 in, 1 out]
            n278 = Fract/Exp String To Number(string=w369) -> (number=w368:dbl)  [unwired: 3 in, 1 out]
            n279 = Bundle(w363, w368) -> (w359:cluster{dbl, dbl})  [unwired: 1 in]
            n280 = Select(t=w353, s=TRUE, f=w359) -> (s? t:f=w358:cluster{dbl, dbl})
            n281 = Build Array(cluster{dbl, dbl} {0.0, 0.0} ("element"), w358) -> (→"joystick":cluster{dbl, dbl}[])
          }
          frame #16 {
            # "System resource"
            n282 = call "fgv_cpu-mem_data.vi"("cmd"=cmd_common."read") -> ("memory out"=w376:dbl, "cpu out"=→"CPU" →"CPU Chart" →"CPU Usage":dbl)  [unwired: 9 in]
            "Mem  Chart" <- w376
            "Mem usage" <- w376
            n283 = Format Into String(format string="%.1f MB", w376) -> (resulting string=→"Mem Usage 2":string)  [unwired: 2 in, 1 out]
            n284 = Multiply(x=w376, y=1000000.0) -> (x*y=→"Mem":dbl)
          }
          frame #17 {
            # "IMU heading"
            n285 = call "fgv_imu_data.vi"("cmd"=cmd_imu."read") -> ("ang"=w387:dbl[], "IMD data out"=→"IMU out":T27)  [unwired: 7 in, 2 out]
            "ang" <- w387
            n286 = local read "Tap_config"() -> (w398:T12)
            n287 = Array To Spreadsheet String(array=w387, 3:"%f" ("포맷 문자열")) -> (spreadsheet string=w384:string)  [unwired: 1 in]
            n288 = call "sub_log_basic.vi"("desc"=w384, "Title"="imu-ang") -> ()  [unwired: 9 in, 1 out]
            n289 = call "fgv_pid_param-var.vi"("cmd"=pid-in-params."read") -> ("pid-var_output"=w390:T56)  [unwired: 10 in]
            n290 = case shown="\"System\", 기본" w398 {
              frame "System", Default {
              }
              frame "AGV" {
              }
              frame "LIDAR" {
              }
              frame "PID" {
              }
              frame "GNSS Gmap" {
              }
              frame "Vision" {
              }
              frame "IMU" {
              }
              frame "File" {
              }
              frame "Waypoint" {
              }
              frame "Joystick" {
              }
              frame "Network" {
              }
              frame "Sound" {
              }
              frame "Etc" {
              }
            }
            n291 = call "fgv_PwrPak7-data.vi"("cmd"=gps-databuf."read") -> ("data cluster out"=w393:T65)  [unwired: 9 in, 1 out]
            n292 = Unbundle By Name(w390) -> ("deg_waypoint"=w389:dbl)
            n293 = Unbundle By Name(w393) -> ("Heading"=w382:dbl)
            "heading_cfg" <- w382
            "heaading_ui" <- w382
            n294 = Subtract(x=w389, y=w382) -> (x-y=→"Deg-gap_heading-wpt":dbl)
            n295 = Equal To 0?(x=w382) -> (x = 0?=w392:bool)
            n296 = call "sub_picture_gnss-deg.vi"("deg_gps"=w382) -> ("new picture"=→"dir":picture)  [unwired: 10 in]
            n297 = flat-sequence {
              tunnel: w392 -> [w400]
              frame #0 {
                n298 = call "sub_error_data-conversion.vi"("error status"=w400) -> ("error conversion out"=w399:u8)  [unwired: 9 in, 1 out]
                n299 = call "fgv_error-2.vi"("cmd"=enum16{"init", "read", "write"}."read") -> ("Error cluster out"=w403:T2)  [unwired: 9 in, 1 out]
                n300 = Bundle By Name(cluster=w403, "Heading"=w399) -> (w404:T2)
                n301 = call "fgv_error-2.vi"("cmd"=enum16{"init", "read", "write"}."write", "Error cluster"=w404) -> ()  [unwired: 8 in, 2 out]
              }
            }
            n302 = Number To Fractional String(number=w382) -> (F-format string=w381:string)  [unwired: 3 in]
            n303 = call "sub_log_basic.vi"("desc"=w381, "Title"="Heading") -> ()  [unwired: 9 in, 1 out]
          }
          frame #18 {
            n304 = call "fgv_timer_buff.vi"("cmd"=enum16{"write", "read"}."read") -> ("time_status out"=w408:T55)  [unwired: 10 in]
            n305 = Unbundle By Name(w408) -> ("total time"=w407:dbl)
            n306 = Number To Fractional String(number=w407, precision (6)=i16 1 ("정밀도(6)")) -> (F-format string=w406:string)  [unwired: 2 in]
            n307 = call "fgv_ledmatrix_config.vi"("cmd"=cmd_common."read") -> ("data out"=w411:T33)  [unwired: 10 in]
            n308 = Bundle By Name(cluster=w411, "time"=w406, "data"=w406) -> (w410:T33)
            n309 = call "fgv_ledmatrix_config.vi"("cmd"=cmd_common."write", "data"=w410) -> ()  [unwired: 9 in, 1 out]
          }
        }
      }
      event "imu reset", "imu reset M": Value Change {
        n310 = event-data() -> ()  [unwired: 1 in, 1 out]
        n311 = call "fgv_imu_data.vi"("cmd"=cmd_imu."ini") -> ()  [unwired: 7 in, 4 out]
      }
      event "SetMapProvider": Value Change {
        n312 = event-data() -> ()  [unwired: 1 in, 1 out]
        n313 = call "fgv_gmap-info.vi"("cmd"=enum16{"read", "write"}."read") -> ("mapinfo 2"=w419:T66)  [unwired: 9 in, 1 out]
        n314 = Unbundle By Name(w419) -> ("mapprovider_info"=w418:T67)
        n315 = Index Array(array=w418, index="SetMapProvider") -> (element=w416:T68)
        n316 = Unbundle By Name(w416) -> ("Name"=w415:string)
        n317 = call "fgv_gmap_core.vi"(7:"cmd"=gmap_fgv-cmd."set map provider" ("cmd"), 10:"cmd"=w415) -> ()  [unwired: 6 in, 4 out]
      }
      event "zoom-center": Value Change {
        n318 = event-data() -> ()  [unwired: 1 in, 1 out]
        n319 = call "fgv_gmap_core.vi"("cmd"=gmap_fgv-cmd."zoom n center markers") -> ()  [unwired: 7 in, 4 out]
      }
      event "Zoom": Value Change {
        n320 = event-data() -> ()  [unwired: 1 in, 1 out]
        n321 = call "fgv_gmap_config.vi"("cmd"=enum16{"read", "write"}."read") -> ("gmap cfg out"=w425:T41)  [unwired: 9 in, 1 out]
        n322 = Bundle By Name(cluster=w425, "zoom n center"="Zoom") -> (w424:T41)
        n323 = call "fgv_gmap_config.vi"("cmd"=enum16{"read", "write"}."write", "gmap cfg"=w424) -> ()  [unwired: 8 in, 2 out]
      }
      event "gmap zoom", "gmap-dt1", "gmap-dt2", "PinDropMrkr": Value Change {
        n324 = event-data() -> ()  [unwired: 1 in, 1 out]
        n325 = local read "Zoom"() -> (w428:bool)
        n326 = Bundle("gmap zoom"="gmap zoom", "gmap-dt1"="gmap-dt1", "gmap-dt2"="gmap-dt2", "PinDropMrkr"="PinDropMrkr", "Zoom"=w428) -> (w431:T69)  [unwired: 1 in]
        n327 = call "fgv_gmap_config.vi"("cmd"=enum16{"read", "write"}."write", "gmap cfg"=w431) -> ()  [unwired: 8 in, 2 out]
      }
      event "Lidar graph scale": Value Change {
        n328 = event-data() -> ()  [unwired: 1 in, 1 out]
        n329 = Negate(x="Lidar graph scale") -> (-x=w435:dbl)
        n330 = property on="LiDAR Display for cfg" class="XYGraph (엄격한)"("XScale.Maximum"="Lidar graph scale", "XScale.Minimum"=w435, "YScale.Maximum"="Lidar graph scale", "YScale.Minimum"=w435) -> ()  [unwired: 2 in, 2 out]
      }
      event "camera_attrib": Value Change {
        n331 = event-data() -> ()  [unwired: 1 in, 1 out]
        n332 = call "sub_camerafile_update.vi"("camera_attrib"="camera_attrib") -> ()  [unwired: 11 in]
      }
      event "Image_gray": Mouse Move {
        n333 = event-data() -> ()  [unwired: 1 in, 1 out]
        n334 = property on="Image_gray" class="ImageControl"() -> ("ROI"=w438:T44)  [unwired: 2 in, 2 out]
        n335 = call "fgv_clamp_roi.vi"("cmd"=enum16{"init", "read", "write"}."write", "ROI-clamp"=w438) -> ()  [unwired: 9 in, 1 out]
      }
      event "camera cfg": Value Change {
        n336 = event-data() -> ()  [unwired: 1 in, 1 out]
        n337 = call "fgv_cam_config.vi"("cmd"=enum16{"read", "write"}."write", "camera cfg"="camera cfg") -> ()  [unwired: 9 in, 1 out]
      }
      event "Vison cfg": Value Change {
        n338 = event-data() -> ()  [unwired: 1 in, 1 out]
        n339 = call "fgv_vision_config.vi"("cmd"=enum16{"init", "read", "write"}."write", "Vison cfg"="Vison cfg") -> ()  [unwired: 8 in, 2 out]
      }
      event "stop points edit": Value Change {
        n340 = event-data() -> ()  [unwired: 1 in, 1 out]
        n341 = flat-sequence {
          frame #0 {
            n342 = call "sub_stop-point_config.vi"() -> ()  [unwired: 12 in]
          }
          frame #1 {
            n343 = call "fgv_waypoint_config.vi"("cmd"=enum16{"read", "write"}."read") -> ("waypoint files cfg out"=w452:T28)  [unwired: 10 in]
            n344 = call "sub_waypoints_upload.vi"("waypoint group"=w452) -> ("waypoint all"=w453:cluster{"XY 그래프":cluster{"X":dbl, "Y":dbl}[]}[])  [unwired: 9 in, 1 out]
            n345 = call "fgv_waypoint_total.vi"("cmd"=enum16{"write", "read"}."write", "waypoint total in"=w453) -> ("waypoint total out"=w451:cluster{"waypt":cluster{"X":dbl, "Y":dbl}[]}[])  [unwired: 9 in]
            n346 = for {
              shift-right: [w455] -> w450
              shift-left: T29 [] -> [w456]
              tunnel: w451 -> [w457] mode=indexing
              n347 = Build Array (concatenate)(w456, w457) -> (w455:cluster{"waypt":cluster{"X":dbl, "Y":dbl}[]}[])
            }
            n348 = call "fgv_stop-point_databuf.vi"("cmd"=enum16{"clear", "write", "read"}."read") -> ("all stop pts out"=w449:cluster{dbl, dbl}[])  [unwired: 9 in, 1 out]
            n349 = Bundle("all stop pts out"=w449) -> (w454:cluster{"all stop pts out":cluster{dbl, dbl}[]})  [unwired: 1 in]
            n350 = Build Array (concatenate)(w454, w450) -> (w444:T29)
            n351 = local write "Total map cfg"(w444) -> ()
          }
        }
      }
      event "stop point config": Value Change {
        n352 = event-data() -> ()  [unwired: 1 in, 1 out]
        n353 = local read "stop point config"() -> (w458:cluster{"distance":dbl, "time":dbl})
        n354 = call "fgv_stop-point_config.vi"("cmd"=enum16{"read", "write"}."write", "config value"=w458) -> ()  [unwired: 9 in, 1 out]
      }
      event "test waypoint": Value Change {
        n355 = event-data() -> ()  [unwired: 1 in, 1 out]
        n356 = flat-sequence {
          frame #0 {
            n357 = disable-structure shown="비활성화" {
              frame Disabled {
                n358 = local read "waypoint files cfg"() -> (w460:T28)
                n359 = call "fgv_waypoint_config.vi"("cmd"=enum16{"read", "write"}."write", "waypoint files cfg"=w460) -> ()  [unwired: 9 in, 1 out]
              }
              frame Enabled {
              }
            }
          }
          frame #1 {
            n360 = call "test_waypoint-files.vi"() -> ()  [unwired: 12 in]
          }
        }
      }
      event "VLP16 cfg": Value Change {
        n361 = event-data() -> ()  [unwired: 1 in, 1 out]
        n362 = call "fgv_lidar-range_vh.vi"("cmd"=enum16{"read", "write"}."write", "VLP16 cfg"="VLP16 cfg") -> ()  [unwired: 9 in, 1 out]
        n363 = case shown="참" FALSE {
          tunnel: "VLP16 cfg" -> [_ w466]
          frame False {
          }
          frame True {
            n364 = Flatten To XML(anything=w466) -> (xml string=w465:string)
            n365 = call "sub_log_basic.vi"("desc"=w465, "Title"="vlp16 cfg  change") -> ()  [unwired: 9 in, 1 out]
          }
        }
      }
      event "RPLidar cfg": Value Change {
        n366 = event-data() -> ()  [unwired: 1 in, 1 out]
        n367 = call "fgv_rplidar_config.vi"("cmd"=enum16{"read", "write"}."write", "RPLidar cfg"="RPLidar cfg") -> ()  [unwired: 8 in, 2 out]
      }
      event Value Change {
        n368 = event-data() -> ()  [unwired: 1 in, 1 out]
        n369 = call "fgv_agv_config.vi"("cmd"=enum16{"read", "write"}."write", "AGV cfg"="AGV cfg") -> ()  [unwired: 8 in, 2 out]
      }
      event "State machine cfg": Value Change {
        n370 = event-data() -> ()  [unwired: 1 in, 1 out]
        n371 = call "fgv_state-machine_config.vi"("cmd"=enum16{"write", "read"}."write", "Angle cfg"="State machine cfg") -> ()  [unwired: 9 in, 1 out]
      }
      event "PID cfg": Value Change {
        n372 = event-data() -> ()  [unwired: 1 in, 1 out]
        n373 = case shown="참" FALSE {
          frame False {
          }
          frame True {
            n374 = call "sub_msgbox.vi"("Reference pid values"=" # Be careful #\n---Ref val--- \np gain: 0.1\nlimit: +- 2000\ndt: 100ms" ("Test title")) -> ()  [unwired: 11 in]
          }
        }
        n375 = call "fgv_pid-config.vi"("cmd"=enum16{"read", "write"}."write", "PID cfg"="PID cfg") -> ()  [unwired: 8 in, 2 out]
      }
      event "waypoint files cfg": Value Change {
        n376 = event-data() -> ()  [unwired: 1 in, 1 out]
        n377 = flat-sequence {
          frame #0 {
            w478 = T29 []
            n378 = call "fgv_waypoint_config.vi"("cmd"=enum16{"read", "write"}."write", "waypoint files cfg"="waypoint files cfg") -> ("waypoint files cfg out"=w485:T28)  [unwired: 9 in]
            n379 = call "sub_waypoints_upload.vi"("waypoint group"=w485) -> ("waypt error"=w479:bool, "waypoint all"=w486:cluster{"XY 그래프":cluster{"X":dbl, "Y":dbl}[]}[])  [unwired: 9 in]
            n380 = call "fgv_waypoint_total.vi"("cmd"=enum16{"write", "read"}."write", "waypoint total in"=w486) -> ("waypoint total out"=w484:cluster{"waypt":cluster{"X":dbl, "Y":dbl}[]}[])  [unwired: 9 in]
            n381 = for {
              shift-right: [w503] -> w482
              shift-left: w478 -> [w504]
              tunnel: w484 -> [w505] mode=indexing
              n382 = Build Array (concatenate)(w504, w505) -> (w503:cluster{"waypt":cluster{"X":dbl, "Y":dbl}[]}[])
            }
            n383 = flat-sequence {
              tunnel: [w490] -> w481
              tunnel: w478 -> [_]
              frame #0 {
                n384 = call "fgv_stop-point_databuf.vi"("cmd"=enum16{"clear", "write", "read"}."read") -> ("all stop pts out"=w490:cluster{dbl, dbl}[])  [unwired: 9 in, 1 out]
              }
            }
            n385 = flat-sequence {
              tunnel: w479 -> [w492]
              frame #0 {
                n386 = call "sub_error_data-conversion.vi"("error status"=w492) -> ("error conversion out"=w493:u8)  [unwired: 9 in, 1 out]
                n387 = call "fgv_error-2.vi"("cmd"=enum16{"init", "read", "write"}."read") -> ("Error cluster out"=w496:T2)  [unwired: 9 in, 1 out]
                n388 = Bundle By Name(cluster=w496, "Waypt"=w493) -> (w497:T2)
                n389 = call "fgv_error-2.vi"("cmd"=enum16{"init", "read", "write"}."write", "Error cluster"=w497) -> ()  [unwired: 8 in, 2 out]
              }
            }
            n390 = case shown="참" TRUE {
              tunnel: [w498 w501] -> w483
              tunnel: w482 -> [w498 w502]
              tunnel: w481 -> [_ w500]
              frame False {
              }
              frame True {
                n391 = Bundle("all stop pts out"=w500) -> (w499:cluster{"all stop pts out":cluster{dbl, dbl}[]})  [unwired: 1 in]
                n392 = Build Array (concatenate)(w499, w502) -> (w501:T29)
              }
            }
            "Total map cfg" <- w483
          }
        }
      }
      event "config load": Value Change {
        n393 = event-data() -> ()  [unwired: 1 in, 1 out]
        n394 = flat-sequence {
          frame #0 {
            n395 = call "fgv_parameter_save-load.vi"("ctl"=T35."Config Load") -> ()  [unwired: 9 in, 2 out]
          }
          frame #1 {
            n396 = call "sub_control-val_update_from_global.vi"() -> ()  [unwired: 12 in]
          }
        }
      }
      event "config save": Value Change {
        n397 = event-data() -> ()  [unwired: 1 in, 1 out]
        n398 = flat-sequence {
          frame #0 {
            n399 = call "sub_control-val_update_to_global.vi"() -> ()  [unwired: 12 in]
          }
          frame #1 {
            n400 = call "fgv_parameter_save-load.vi"("ctl"=T35."Config Save", "file name"="config_file-name") -> ()  [unwired: 8 in, 2 out]
          }
        }
      }
      event "Checking": Value Change {
        n401 = event-data() -> ()  [unwired: 1 in, 1 out]
        n402 = call "fgv_hw-info.vi"("cmd"=enum16{"write", "read"}."read") -> ("HW info out"=w518:T13)  [unwired: 10 in]
        n403 = Unbundle(w518) -> ("AGV"=w517:enum16{"none", "ERP42", "Scout", "Ycar"}, "Lidar 1"=w516:T70, "Lidar 2"=w515:T70, "GPS"=w514:T71, "Camera"=w513:T72, "Joystick"=w512:enum16{"none", "joystick"}, "sound"=w510:enum16{"none", "speaker"}, "IMU"=w511:enum16{"none", "MW-AHRSv1"}, "Led"=w509:enum16{"none", "LedMatrix 8x32"})
        n404 = stacked-sequence {
          tunnel: w517 -> [w523 _ _ _ _ _ _ _ _]
          tunnel: w516 -> [_ w530 _ _ _ _ _ _ _]
          tunnel: w515 -> [_ _ w537 _ _ _ _ _ _]
          tunnel: w514 -> [_ _ _ w538 _ _ _ _ _]
          tunnel: w513 -> [_ _ _ _ w543 _ _ _ _]
          tunnel: w512 -> [_ _ _ _ _ w546 _ _ _]
          tunnel: w511 -> [_ _ _ _ _ _ _ w554 _]
          tunnel: w510 -> [_ _ _ _ _ _ w549 _ _]
          tunnel: w509 -> [_ _ _ _ _ _ _ _ w557]
          frame #0 {
            n405 = case shown="\"Scout\"" w523 {
              frame "ERP42" {
                n406 = call "fgv_erp42_q.vi"("cmd"=enum16{"create", "write", "read", "close"}."write", "data"=enum16{"run", "check", "stop"}."check") -> ()  [unwired: 8 in, 2 out]
              }
              frame "Scout" {
                n407 = call "fgv_q_agv.vi"("cmd"=enum16{"create", "write", "read", "close"}."write", "data"=enum16{"run", "check", "stop"}."check") -> ()  [unwired: 8 in, 2 out]
              }
              frame "Ycar" {
                n408 = call "fgv_ycar_q.vi"("cmd"=enum16{"create", "write", "read", "close"}."write", "data"=enum16{"run", "check", "stop"}."check") -> ()  [unwired: 8 in, 2 out]
              }
              frame "none", Default {
              }
            }
          }
          frame #1 {
            n409 = case shown="\"none\", 기본" w530 {
              frame "none", Default {
              }
              frame "VLP16" {
                n410 = call "fgv_q_vlp16.vi"("cmd"=enum16{"create", "write", "read", "close"}."write", "data"=enum16{"run", "check", "stop"}."check") -> ()  [unwired: 8 in, 2 out]
              }
              frame "TIM571" {
                n411 = call "fgv_q_tim571.vi"("cmd"=enum16{"create", "write", "read", "close"}."write", "data"=enum16{"run", "check", "stop"}."check") -> ()  [unwired: 8 in, 2 out]
              }
              frame "RPLidar A2", "RPLidar A3" {
                n412 = call "fgv_rplidar_232_q.vi"("cmd"=enum16{"create", "write", "read", "close"}."write", "data"=enum16{"run", "check", "stop"}."check") -> ()  [unwired: 8 in, 2 out]
              }
            }
          }
          frame #2 {
            n413 = case shown="\"none\", 기본" w537 {
              frame "none", Default {
              }
              frame "VLP16" {
              }
            }
          }
          frame #3 {
            n414 = case shown="\"F9P\", \"M8P\"" w538 {
              frame "none", Default {
              }
              frame "F9P", "M8P" {
                n415 = call "fgv_F9P_q.vi"("cmd"=enum16{"create", "write", "read", "close"}."write", "data"=enum16{"run", "check", "stop"}."check") -> ()  [unwired: 8 in, 2 out]
              }
              frame "PwrPak7" {
                n416 = call "fgv_q_PwrPak7.vi"("cmd"=enum16{"create", "write", "read", "close"}."write", "data"=enum16{"run", "check", "stop"}."check") -> ()  [unwired: 8 in, 2 out]
              }
              frame "19X HVS" {
              }
            }
          }
          frame #4 {
            # "Cam"
            n417 = case shown="\"C920\", 기본" w543 {
              frame "none" {
              }
              frame "C920", Default {
                n418 = call "fgv_pc_cam_q.vi"("cmd"=enum16{"create", "write", "read", "close"}."write", "data"=enum16{"run", "check", "stop"}."check") -> ()  [unwired: 8 in, 2 out]
              }
            }
          }
          frame #5 {
            # "joystick"
            n419 = case shown="\"joystick\", 기본" w546 {
              frame "none" {
              }
              frame "joystick", Default {
                n420 = call "fgv_q_joystick.vi"("cmd"=enum16{"create", "write", "read", "close"}."write", "data"=enum16{"run", "check", "stop"}."check") -> ()  [unwired: 8 in, 2 out]
              }
            }
          }
          frame #6 {
            n421 = case shown="\"speaker\"" w549 {
              frame "none", Default {
              }
              frame "speaker" {
                n422 = Bundle(cluster=T54 {"FN"=enum."music", "Data"=variant} ("data"), "FN"=T53."unlock") -> (w553:T54)  [unwired: 1 in]
                n423 = call "fgv_sound_q.vi"("cmd"=enum16{"create", "write", "read", "close"}."write", "data"=w553) -> ()  [unwired: 8 in, 2 out]
              }
            }
          }
          frame #7 {
            # "joystick"
            n424 = case shown="\"MW-AHRSv1\"" w554 {
              frame "none", Default {
              }
              frame "MW-AHRSv1" {
                n425 = call "fgv_imu_q_pro-con.vi"("cmd"=enum16{"create", "write", "read", "close"}."write", "data"=enum16{"run", "check", "stop"}."check") -> ()  [unwired: 8 in, 2 out]
              }
            }
          }
          frame #8 {
            n426 = case shown="\"LedMatrix 8x32\"" w557 {
              frame "none", Default {
              }
              frame "LedMatrix 8x32" {
                n427 = call "fgv_ledmatrix_q.vi"("cmd"=enum16{"create", "write", "read", "close"}."write", "data"=enum16{"run", "check", "stop"}."check") -> ()  [unwired: 8 in, 2 out]
              }
            }
          }
        }
        n428 = property on="start-stop" class="Bool (엄격한)"("DisabledEnum"=T38."Enabled" ("비활성화")) -> ()  [unwired: 2 in, 2 out]
        n429 = call "fgv_status-display.vi"("Mode"=enum16{"Initial", "Update", "Clear"}."Update", "title"="*** HW checking ***" ("String in 1")) -> ()  [unwired: 9 in, 1 out]
      }
      event "LiDAR Display": Mouse Down {
        n430 = event-data() -> ()  [unwired: 1 in, 1 out]
      }
      event "state change": Value Change {
        n431 = event-data() -> ()  [unwired: 1 in, 1 out]
        n432 = call "fgv_system_state.vi"("cmd"=enum16{"init", "read", "write"}."write", "State"="set state value") -> ("State out"=w560:T3)  [unwired: 8 in, 1 out]
        n433 = flat-sequence {
          tunnel: w560 -> [_]
          frame #0 {
            n434 = call "fgv_loop_count.vi"("cmd"=enum16{"init", "read", "write"}."read") -> ()  [unwired: 9 in, 2 out]
          }
        }
      }
      event "Lookahead cfg": Value Change {
        n435 = event-data() -> ()  [unwired: 1 in, 1 out]
        n436 = call "fgv_look-ahead_config.vi"("cmd"=enum16{"read", "write"}."write", "lookahed cfg in"="Lookahead cfg") -> ()  [unwired: 9 in, 1 out]
      }
      event "start-stop": Value Change {
        n437 = event-data() -> ()  [unwired: 1 in, 1 out]
        n438 = case shown="참" "start-stop" {
          frame False {
            n439 = call "fgv_local-stop_agv.vi"("cmd"=enum16{"ini", "read", "stop"}."stop") -> ()  [unwired: 10 in, 1 out]
            n440 = property on="Checking" class="Bool"("DisabledEnum"=T38."Enabled" ("비활성화")) -> ()  [unwired: 2 in, 2 out]
            n441 = call "sub_system_pause-condition.vi"("cmd"=enum16{"pause", "go", "read"}."pause") -> ()  [unwired: 10 in, 1 out]
            n442 = disable-structure shown="비활성화" {
              frame Disabled {
                n443 = property on="start-stop" class="Bool (엄격한)" props=["DisabledEnum"]() -> ()  [unwired: 3 in, 2 out]
              }
              frame Enabled {
              }
            }
            n444 = call "fgv_status-display.vi"("Mode"=enum16{"Initial", "Update", "Clear"}."Update", "detail"="----Stop----", "title"="" ("String in 1")) -> ()  [unwired: 8 in, 1 out]
          }
          frame True {
            n445 = flat-sequence {
              frame #0 {
                n446 = call "fgv_local-stop_agv.vi"("cmd"=enum16{"ini", "read", "stop"}."ini") -> ()  [unwired: 10 in, 1 out]
                n447 = call "sub_system_pause-condition.vi"("cmd"=enum16{"pause", "go", "read"}."go") -> ()  [unwired: 10 in, 1 out]
              }
              frame #1 {
                n448 = call "fgv_hw-info.vi"("cmd"=enum16{"write", "read"}."read") -> ("HW info out"=w585:T13)  [unwired: 10 in]
                n449 = Unbundle(w585) -> ("AGV"=w584:enum16{"none", "ERP42", "Scout", "Ycar"}, "Lidar 1"=w583:T70, "Lidar 2"=w582:T70, "GPS"=w581:T71, "Camera"=w580:T72, "Joystick"=w578:enum16{"none", "joystick"}, "sound"=w577:enum16{"none", "speaker"}, "IMU"=w576:enum16{"none", "MW-AHRSv1"}, "Led"=w575:enum16{"none", "LedMatrix 8x32"})
                n450 = stacked-sequence {
                  tunnel: w584 -> [w586 _ _ _ _ _ _ _ _ _]
                  tunnel: w583 -> [_ w593 _ _ _ _ _ _ _ _]
                  tunnel: w582 -> [_ _ w600 _ _ _ _ _ _ _]
                  tunnel: w581 -> [_ _ _ w601 _ _ _ _ _ _]
                  tunnel: w580 -> [_ _ _ _ w606 _ _ _ _ _]
                  tunnel: w578 -> [_ _ _ _ _ _ w609 _ _ _]
                  tunnel: w577 -> [_ _ _ _ _ _ _ w612 _ _]
                  tunnel: w576 -> [_ _ _ _ _ _ _ _ w617 _]
                  tunnel: w575 -> [_ _ _ _ _ _ _ _ _ w620]
                  frame #0 {
                    n451 = case shown="\"Scout\"" w586 {
                      frame "ERP42" {
                        n452 = call "fgv_erp42_q.vi"("cmd"=enum16{"create", "write", "read", "close"}."write", "data"=enum16{"run", "check", "stop"}."run") -> ()  [unwired: 8 in, 2 out]
                      }
                      frame "Scout" {
                        n453 = call "fgv_q_agv.vi"("cmd"=enum16{"create", "write", "read", "close"}."write", "data"=enum16{"run", "check", "stop"}."run") -> ()  [unwired: 8 in, 2 out]
                      }
                      frame "Ycar" {
                        n454 = call "fgv_ycar_q.vi"("cmd"=enum16{"create", "write", "read", "close"}."write", "data"=enum16{"run", "check", "stop"}."run") -> ()  [unwired: 8 in, 2 out]
                      }
                      frame "none", Default {
                      }
                    }
                  }
                  frame #1 {
                    n455 = case shown="\"TIM571\"" w593 {
                      frame "none", Default {
                      }
                      frame "VLP16" {
                        n456 = call "fgv_q_vlp16.vi"("cmd"=enum16{"create", "write", "read", "close"}."write", "data"=enum16{"run", "check", "stop"}."run") -> ()  [unwired: 8 in, 2 out]
                      }
                      frame "TIM571" {
                        n457 = call "fgv_q_tim571.vi"("cmd"=enum16{"create", "write", "read", "close"}."write", "data"=enum16{"run", "check", "stop"}."run") -> ()  [unwired: 8 in, 2 out]
                      }
                      frame "RPLidar A2", "RPLidar A3" {
                        n458 = call "fgv_rplidar_232_q.vi"("cmd"=enum16{"create", "write", "read", "close"}."write", "data"=enum16{"run", "check", "stop"}."run") -> ()  [unwired: 8 in, 2 out]
                      }
                    }
                  }
                  frame #2 {
                    n459 = case shown="\"TIM571\"" w600 {
                      frame "none", Default {
                      }
                      frame "VLP16" {
                      }
                      frame "TIM571" {
                      }
                      frame "RPLidar A2" {
                      }
                      frame "RPLidar A3" {
                      }
                    }
                  }
                  frame #3 {
                    n460 = case shown="\"F9P\", \"M8P\"" w601 {
                      frame "none", Default {
                      }
                      frame "F9P", "M8P" {
                        n461 = call "fgv_F9P_q.vi"("cmd"=enum16{"create", "write", "read", "close"}."write", "data"=enum16{"run", "check", "stop"}."run") -> ()  [unwired: 8 in, 2 out]
                      }
                      frame "PwrPak7" {
                        n462 = call "fgv_q_PwrPak7.vi"("cmd"=enum16{"create", "write", "read", "close"}."write", "data"=enum16{"run", "check", "stop"}."run") -> ()  [unwired: 8 in, 2 out]
                      }
                      frame "19X HVS" {
                      }
                    }
                  }
                  frame #4 {
                    n463 = case shown="\"C920\", 기본" w606 {
                      frame "none" {
                      }
                      frame "C920", Default {
                        n464 = call "fgv_pc_cam_q.vi"("cmd"=enum16{"create", "write", "read", "close"}."write", "data"=enum16{"run", "check", "stop"}."run") -> ()  [unwired: 8 in, 2 out]
                      }
                    }
                  }
                  frame #5 {
                    # "joystick / useless"
                  }
                  frame #6 {
                    n465 = case shown="\"joystick\"" w609 {
                      frame "none", Default {
                      }
                      frame "joystick" {
                        n466 = call "fgv_q_joystick.vi"("cmd"=enum16{"create", "write", "read", "close"}."write", "data"=enum16{"run", "check", "stop"}."run") -> ()  [unwired: 8 in, 2 out]
                      }
                    }
                  }
                  frame #7 {
                    n467 = case shown="\"speaker\"" w612 {
                      frame "none", Default {
                      }
                      frame "speaker" {
                        n468 = Bundle(cluster=T54 {"FN"=enum."music", "Data"=variant} ("data"), "FN"=T53."engine") -> (w616:T54)  [unwired: 1 in]
                        n469 = call "fgv_sound_q.vi"("cmd"=enum16{"create", "write", "read", "close"}."write", "data"=w616) -> ()  [unwired: 8 in, 2 out]
                      }
                    }
                  }
                  frame #8 {
                    n470 = case shown="\"MW-AHRSv1\"" w617 {
                      frame "none", Default {
                      }
                      frame "MW-AHRSv1" {
                        n471 = call "fgv_imu_q_pro-con.vi"("cmd"=enum16{"create", "write", "read", "close"}."write", "data"=enum16{"run", "check", "stop"}."run") -> ()  [unwired: 8 in, 2 out]
                      }
                    }
                  }
                  frame #9 {
                    n472 = case shown="\"LedMatrix 8x32\"" w620 {
                      frame "none", Default {
                      }
                      frame "LedMatrix 8x32" {
                        n473 = call "fgv_ledmatrix_q.vi"("cmd"=enum16{"create", "write", "read", "close"}."write", "data"=enum16{"run", "check", "stop"}."run") -> ()  [unwired: 8 in, 2 out]
                      }
                    }
                  }
                }
              }
              frame #2 {
                n474 = property on="pause-resume" class="Bool (엄격한)"("DisabledEnum"=T38."Enabled" ("비활성화")) -> ()  [unwired: 2 in, 2 out]
                n475 = property on="Checking" class="Bool"("DisabledEnum"=T38."Disabled and Grayed Out" ("비활성화")) -> ()  [unwired: 2 in, 2 out]
                n476 = call "fgv_status-display.vi"("Mode"=enum16{"Initial", "Update", "Clear"}."Update", "detail"="----Start----", "title"="" ("String in 1")) -> ()  [unwired: 8 in, 1 out]
              }
            }
          }
        }
      }
      event Value Change {
        n477 = event-data() -> ()  [unwired: 1 in, 1 out]
        n478 = call "fgv_ledmatrix_config.vi"("cmd"=cmd_common."write", "data"="ledmatrix cfg") -> ()  [unwired: 9 in, 1 out]
      }
      event Value Change {
        n479 = event-data() -> ()  [unwired: 1 in, 1 out]
        n480 = call "fgv_imu_config.vi"("cmd"=enum16{"read", "write"}."write", "IMU cfg"="IMU cfg") -> ()  [unwired: 8 in, 2 out]
      }
      event Value Change {
        n481 = event-data() -> ()  [unwired: 1 in, 1 out]
        n482 = call "fgv_gps_config.vi"("cmd"=enum16{"read", "write"}."write", "GNSS cfg"="GNSS cfg") -> ()  [unwired: 8 in, 2 out]
      }
      event Value Change {
        n483 = event-data() -> ()  [unwired: 1 in, 1 out]
        n484 = call "fgv_joystick_config.vi"("cmd"=cmd_common."write", "Joystick cfg"="Joystick cfg") -> ("Joystick cfg out"=w641:T30)  [unwired: 8 in, 1 out]
        n485 = Unbundle By Name(w641) -> ("steer limit.min"=w639:dbl, "steer limit.max"=w640:dbl)  [unwired: 2 out]
        n486 = Subtract(x=w640, y=w639) -> (x-y=w638:dbl)
        n487 = Divide(x=w638, y=2.0) -> (x/y=w636:dbl)
        n488 = Negate(x=w636) -> (-x=w635:dbl)
        n489 = Bundle(w636, w635) -> (→"pid limit ref":cluster{dbl, dbl})  [unwired: 1 in]
      }
      event "sel driving mode": Value Change {
        n490 = event-data() -> ()  [unwired: 1 in, 1 out]
        n491 = call "fgv_control-select.vi"("cmd"=cmd_common."write", "mode"=enum16{"joystick", "self-driving"}."self-driving") -> ()  [unwired: 9 in, 1 out]
      }
      event "Speed": Value Change {
        n492 = event-data() -> ()  [unwired: 1 in, 1 out]
        n493 = flat-sequence {
          tunnel: "Speed" -> [w649]
          frame #0 {
            n494 = call "fgv_agv_speedsteer-common.vi"("cmd"=enum16{"init", "read", "write"}."read") -> ("speed-steer out"=w648:cluster{"speed":dbl, "steer":dbl})  [unwired: 10 in]
            n495 = Bundle By Name(cluster=w648, "speed"=w649) -> (w647:cluster{"speed":dbl, "steer":dbl})
            n496 = call "fgv_agv_speedsteer-common.vi"("cmd"=enum16{"init", "read", "write"}."write", "speed-steer"=w647) -> ()  [unwired: 9 in, 1 out]
          }
        }
      }
      event Value Change {
        n497 = event-data() -> ()  [unwired: 1 in, 1 out]
        n498 = call "fgv_hw-info.vi"("cmd"=enum16{"write", "read"}."write", "HW info"="HW info") -> ()  [unwired: 9 in, 1 out]
      }
      event "Obstacle limit cfg": Value Change {
        n499 = event-data() -> ()  [unwired: 1 in, 1 out]
        n500 = call "fgv_obstacle_data.vi"("cmd"=obstacle_info."write limit", "limit in"="Obstacle limit cfg") -> ()  [unwired: 6 in, 4 out]
      }
      event "close": Value Change {
        n501 = event-data() -> ()  [unwired: 1 in, 1 out]
        n502 = flat-sequence {
          tunnel: [w660] -> w656
          tunnel: [w677] -> w657
          tunnel: w656 -> [w677]
          frame #0 {
            n503 = stacked-sequence {
              frame #0 {
                n504 = call "fgv_ycar_q.vi"("cmd"=enum16{"create", "write", "read", "close"}."close") -> ()  [unwired: 9 in, 2 out]
              }
              frame #1 {
                n505 = call "fgv_rplidar_232_q.vi"("cmd"=enum16{"create", "write", "read", "close"}."close") -> ()  [unwired: 9 in, 2 out]
              }
              frame #2 {
                n506 = call "fgv_q_joystick.vi"("cmd"=enum16{"create", "write", "read", "close"}."close") -> ()  [unwired: 9 in, 2 out]
              }
              frame #3 {
                n507 = call "fgv_sound_q.vi"("cmd"=enum16{"create", "write", "read", "close"}."close") -> ()  [unwired: 9 in, 2 out]
              }
              frame #4 {
                n508 = call "fgv_logbuff_q.vi"("cmd"=log_buffq."close") -> ()  [unwired: 9 in, 2 out]
              }
              frame #5 {
                n509 = call "fgv_imu_q_pro-con.vi"("cmd"=enum16{"create", "write", "read", "close"}."close") -> ()  [unwired: 9 in, 2 out]
              }
              frame #6 {
                n510 = call "fgv_pc_cam_q.vi"("cmd"=enum16{"create", "write", "read", "close"}."close") -> ()  [unwired: 9 in, 2 out]
              }
              frame #7 {
                n511 = call "fgv_F9P_q.vi"("cmd"=enum16{"create", "write", "read", "close"}."close") -> ()  [unwired: 9 in, 2 out]
              }
              frame #8 {
                n512 = call "fgv_ledmatrix_q.vi"("cmd"=enum16{"create", "write", "read", "close"}."close") -> ()  [unwired: 9 in, 2 out]
              }
            }
            n513 = case shown="거짓" TRUE {
              frame False {
                n514 = stacked-sequence {
                  frame #0 {
                    n515 = call "fgv_q_agv.vi"("cmd"=enum16{"create", "write", "read", "close"}."close") -> ()  [unwired: 9 in, 2 out]
                  }
                  frame #1 {
                    n516 = call "fgv_erp42_q.vi"("cmd"=enum16{"create", "write", "read", "close"}."close") -> ()  [unwired: 9 in, 2 out]
                  }
                  frame #2 {
                    n517 = call "fgv_erp42mini-232_q.vi"("cmd"=enum16{"create", "write", "read", "close"}."close") -> ()  [unwired: 9 in, 2 out]
                  }
                  frame #3 {
                    n518 = call "fgv_q_PwrPak7.vi"("cmd"=enum16{"create", "write", "read", "close"}."close") -> ()  [unwired: 9 in, 2 out]
                  }
                  frame #4 {
                    n519 = call "fgv_q_vlp16.vi"("cmd"=enum16{"create", "write", "read", "close"}."close") -> ()  [unwired: 9 in, 2 out]
                  }
                  frame #5 {
                    n520 = call "fgv_q_tim571.vi"("cmd"=enum16{"create", "write", "read", "close"}."close") -> ()  [unwired: 9 in, 2 out]
                  }
                }
              }
              frame True {
              }
            }
            n521 = call "fgv_global-stop.vi"("cmd"=enum16{"init", "stop", "read"}."stop") -> ("val_out"=w660:bool)  [unwired: 10 in]
          }
          frame #1 {
            n522 = local write "close"(FALSE ("close")) -> ()
          }
        }
      }
      event "sound cfg": Value Change {
        n523 = event-data() -> ()  [unwired: 1 in, 1 out]
        n524 = call "fgv_sound_config.vi"("cmd"=cmd_common."write", "data"="sound cfg") -> ()  [unwired: 9 in, 1 out]
      }
      event "pause-resume": Value Change {
        n525 = event-data() -> ()  [unwired: 1 in, 1 out]
        n526 = case shown="거짓" "pause-resume" {
          frame False {
            n527 = call "sub_system_pause-condition.vi"("cmd"=enum16{"pause", "go", "read"}."go") -> ()  [unwired: 10 in, 1 out]
            n528 = call "fgv_status-display.vi"("Mode"=enum16{"Initial", "Update", "Clear"}."Update", "title"="----Go----" ("String in 1")) -> ()  [unwired: 9 in, 1 out]
          }
          frame True {
            n529 = call "sub_system_pause-condition.vi"("cmd"=enum16{"pause", "go", "read"}."pause") -> ()  [unwired: 10 in, 1 out]
            n530 = call "fgv_status-display.vi"("Mode"=enum16{"Initial", "Update", "Clear"}."Update", "title"="----Pause----" ("String in 1")) -> ()  [unwired: 9 in, 1 out]
          }
        }
      }
      event "TIM571 cfg": Value Change {
        n531 = event-data() -> ()  [unwired: 1 in, 1 out]
        n532 = call "fgv_tim571_setting.vi"("cmd"=enum16{"write", "read"}."write", "tim571_setting-data_in"="TIM571 cfg") -> ()  [unwired: 9 in, 1 out]
      }
    }
  }
  n533 = call "sub_main_gmap.vi"("error in"=w6) -> ("error out"=w5:errorcluster)  [unwired: 10 in]
  n534 = Merge Errors(w30, w29, w28, w27, w21, w20, w5) -> (w19:errorcluster)
  n535 = call "sub_cam_main.vi"("error in"=w2) -> ("error out"=w26:errorcluster)  [unwired: 10 in]
  n536 = call "sub_main_vision.vi"("error in"=w2) -> ("error out"=w25:errorcluster)  [unwired: 10 in]
  n537 = call "sub_main_timer.vi"("error in"=w2) -> ("error out"=w24:errorcluster)  [unwired: 10 in]
  n538 = call "sub_main_data-process.vi"("error in"=w2) -> ("error out"=w23:errorcluster)  [unwired: 10 in]
  n539 = call "sub_main_pid.vi"("error in"=w2) -> ("error out"=w15:errorcluster)  [unwired: 10 in]
  n540 = call "sub_main_speed-control.vi"("error in"=w2) -> ("error out"=w16:errorcluster)  [unwired: 10 in]
  n541 = call "sub_main_state.vi"("error in"=w2) -> ("error out"=w17:errorcluster)  [unwired: 10 in]
  n542 = call "sub_main_appcomm.vi"("error in"=w2) -> ("error out"=w18:errorcluster)  [unwired: 10 in]
  n543 = call "sub_main_joystick.vi"("error in"=w2) -> ("error out"=w13:errorcluster)  [unwired: 10 in]
  n544 = Merge Errors(w26, w25, w24, w23, w15, w16, w17, w18, w13) -> (w14:errorcluster)
  n545 = call "sub_rplidar_main.vi"("error in"=w2) -> ("error out"=w12:errorcluster)  [unwired: 10 in]
  n546 = call "sub_main_ycar.vi"("error in"=w2) -> ("error out"=w11:errorcluster)  [unwired: 10 in]
  n547 = call "sub_main_imu.vi"("error in"=w2) -> ("error out"=w3:errorcluster)  [unwired: 10 in]
  n548 = call "sub_main_cpu-memroy_usage.vi"("error in"=w2) -> ("error out"=w9:errorcluster)  [unwired: 10 in]
  n549 = call "sub_main_sound.vi"("error in"=w2) -> ("error out"=w8:errorcluster)  [unwired: 10 in]
  n550 = call "sub_main_Nstream.vi"("error in"=w2) -> ("error out"=w7:errorcluster)  [unwired: 10 in]
  n551 = call "sub_main_ledmatrix.vi"("error in"=w2) -> ("error out"=w1:errorcluster)  [unwired: 10 in]
  n552 = Merge Errors(w12, w11, w3, w9, w8, w7, w1) -> (w4:errorcluster)
  n553 = disable-structure shown="비활성화" {
    disable-tunnel: w4 -> [w689 _]
    frame Disabled {
      n554 = call "sub_main_pwrpak7.vi"("error in"=w689) -> ()  [unwired: 10 in, 1 out]
      n555 = call "sub_main_agv.vi"("error in"=w689) -> ()  [unwired: 10 in, 1 out]
    }
    frame Enabled {
    }
  }
  n556 = flat-sequence {
    tunnel: w32 -> [_]
    tunnel: [w690] -> w31
    frame #0 {
      n557 = call "fgv_status-display.vi"("Mode"=enum16{"Initial", "Update", "Clear"}."Update", "title"="Producer fihish" ("String in 1")) -> ("error out"=w690:errorcluster)  [unwired: 9 in]
    }
  }
  n558 = Merge Errors(w4, w14, w19) -> (w22:errorcluster)
  n559 = flat-sequence {
    tunnel: w31 -> [_]
    tunnel: w22 -> [_]
    frame #0 {
      n560 = call "sub_update-parameters-to-global for save.vi"() -> ()  [unwired: 12 in]
    }
    frame #1 {
      n561 = call "sub_control-val_update_to_global.vi"() -> ()  [unwired: 12 in]
    }
    frame #2 {
      n562 = call "fgv_parameter_save-load.vi"("ctl"=T35."LastRUN Save") -> ()  [unwired: 9 in, 2 out]
      n563 = call "fgv_lidars-img.vi"("cmd"=enum16{"create", "read", "close"}."close") -> ()  [unwired: 10 in, 1 out]
      n564 = call "sub_register-event-callback.vi"("cmd"=enum16{"register", "close"}."close") -> ("error out"=w693:errorcluster)  [unwired: 10 in]
      n565 = call "fgv_gmap_core.vi"("cmd"=gmap_fgv-cmd."close", "error in"=w693) -> ()  [unwired: 6 in, 4 out]
      n566 = call "fgv_status-display.vi"("Mode"=enum16{"Initial", "Update", "Clear"}."Update", "title"="Shut down" ("String in 1")) -> ()  [unwired: 9 in, 1 out]
    }
    frame #3 {
      n567 = case shown="거짓" FALSE {
        frame False {
        }
        frame True {
          n568 = call "IMAQ Dispose"("All Images? (No)"=TRUE) -> ()  [unwired: 5 in, 1 out]
        }
      }
      n569 = local write "close"(FALSE ("stop")) -> ()
    }
  }
